vi "DOCK_AUDIT_MAIN.vi"() -> ()   [LabVIEW 2020]
uses:
  DOCK_AUDIT/MAIN/DOCK_header_data_display.ctl
  DOCK_AUDIT/FGV/error_buffer/FGV_DOCK_error_buffer.ctl
  DOCK_AUDIT/ini/typedef/DOCK_all_config_info.ctl
  DOCK_AUDIT/ini/typedef/DOCK_main_ini_file.ctl
  DOCK_AUDIT/queues/typedef/DOCK_queue_refnums.ctl
  DOCK_AUDIT/queues/typedef/DOCK_MAIN_queue_element.ctl
  DOCK_AUDIT/MAIN/DOCK_MAIN_sequence_state.ctl
  DOCK_AUDIT/queues/typedef/DOCK_SCANNER_queue_element.ctl
  DOCK_AUDIT/SCANNER/DOCK_SCANNER_sequence_state.ctl
  DOCK_AUDIT/queues/typedef/DOCK_PRINTER_queue_element.ctl
  DOCK_AUDIT/PRINTER/DOCK_PRINTER_sequence_state.ctl
  DOCK_AUDIT/FGV/SQL_connection/FGV_DOCK_SQL_connection.ctl
  DOCK_AUDIT/FGV/login/DOCK_login_refnums.ctl
  DOCK_AUDIT/FGV/login/FGV_DOCK_login.ctl
  DOCK_AUDIT/FGV/DOCK_status_display/FGV_DOCK_status_display.ctl
  DOCK_AUDIT/FGV/DOCK_records_display/FGV_DOCK_records_display.ctl
  DOCK_AUDIT/FGV/DOCK_records_display/DOCK_references.ctl
  DOCK_AUDIT/FGV/controls_state/FGV_DOCK_controls_state.ctl
  DOCK_AUDIT/FGV/controls_state/FGV_DOCK_controls_state_refnums.ctl
  DOCK_AUDIT/FGV/DOCK_batch_ID_buffer/FGV_DOCK_batch_ID_buffer.ctl
  DOCK_AUDIT/FGV/DOCK_multistate_indicator/FGV_DOCK_multistate_indicator.ctl
  DOCK_AUDIT/FGV/DOCK_REPORT_records_display/FGV_DOCK_REPORT_records_display.ctl
  DOCK_AUDIT/FGV/DOCK_REPORT_records_display/DOCK_REPORT_references.ctl
  DOCK_AUDIT/FGV/DOCK_REPORT_status_display/FGV_DOCK_REPORT_status_display.ctl
  DOCK_AUDIT/MAIN/DOCK_thread.ctl
  DOCK_AUDIT/ini/typedef/DOCK_reload_data.ctl
  DOCK_AUDIT/FGV/config_info/FGV_DOCK_config_info.ctl
  _misc/AULocalize/SubVIs/RegisterVI.vi
  <vilib>/Instr/_visa.llb/VISA Configure Serial Port (Instr).vi
  _misc/AULocalize/SubVIs/Get Localized Phrase Compact Interface 1D.vi
  _misc/AULocalize/SubVIs/Get Localized Phrase Compact Interface 0D.vi
panel:
  out "app_title":string caption="A603 - Dock Audit"
  in  "reload_reference_data":bool
  in  "print_label_test":bool
  out "reload_active?":bool
  out "reload_batch_size":u16 caption="Размер партии:"
  out "reload_part_number":string caption="Номер партии:"
  in  "printer_send_label":bool
  in  "printer_send_template":bool
  out "current_batch_count":u16 caption="В текущей партии:"
  out "batch_active?":bool
  out "PRINTER_connection_indicator_global":bool caption="Статус подключения принтера:"
  in  "DOCK_start_finish_batch":bool
  in  "BATCH_SIZE_selector":u16(ring)=30 caption="Размер партии:" items=["36"=36, "30"=30, "10"=10, "6"=6, "1"=1]
  in  "REFERENCE_selector":u16(ring) caption="Тип детали:" items=["CMFB", "VESTA"]
  in  "USER_login_logout":bool
  out "SQL_connection_indicator_global":bool caption="Статус подключения SQL:"
  out "ERROR_indicator_global":bool caption="Статус программы:"
  out "current_access_level":i32 caption="Уровень доступа:"
  out "current_username":string="-" caption="Вход под ID:"
  in  "main_tab":enum32{"Dock Audit", "Current Batch", "Errors"}(tab)=enum."Errors"
  out "gear_serial_display":string
  in  "gear_NOK":bool
  in  "gear_OK":bool
  in  "DOCK_clear_gear_data":bool
  out "DOCK_multistate_indicator":bool=TRUE
  in  "DOCK_read_gear_data":bool
  in  "DOCK_records":i32(listbox)=-1
  out "DOCK_SQL_status":string="READ BATCH SIZE LIST - OK\nExecuted SQL statement: SELECT DISTINCT BATCH_SIZE FROM DOCK_AUDIT_BATCH_SIZE ORDER BY BATCH_SIZE DESC"
  in  "DOCK_gear_serial":string caption="Номер детали:"
  out "batch_code_display":string
  out "DOCK_header_data_display":T1
  out "input_header":string caption="Вход"
  out "gear_info_summary_header":string caption="Информация о детали"
  in  "REPORT_clear":bool
  in  "REPORT_records":i32(listbox)=-1
  out "DOCK_REPORT_SQL_status":string="READ BATCH SIZE LIST - OK\nExecuted SQL statement: SELECT DISTINCT BATCH_SIZE FROM DOCK_AUDIT_BATCH_SIZE ORDER BY BATCH_SIZE DESC"
  in  "REPORT_reload":bool
  out "REPORT_current_batch":string
  in  "ERROR_records":i32(listbox)=-1
  in  "ERROR_clear":bool
  out "ERROR_indicator_tab":bool
  in  "STOP":bool=TRUE
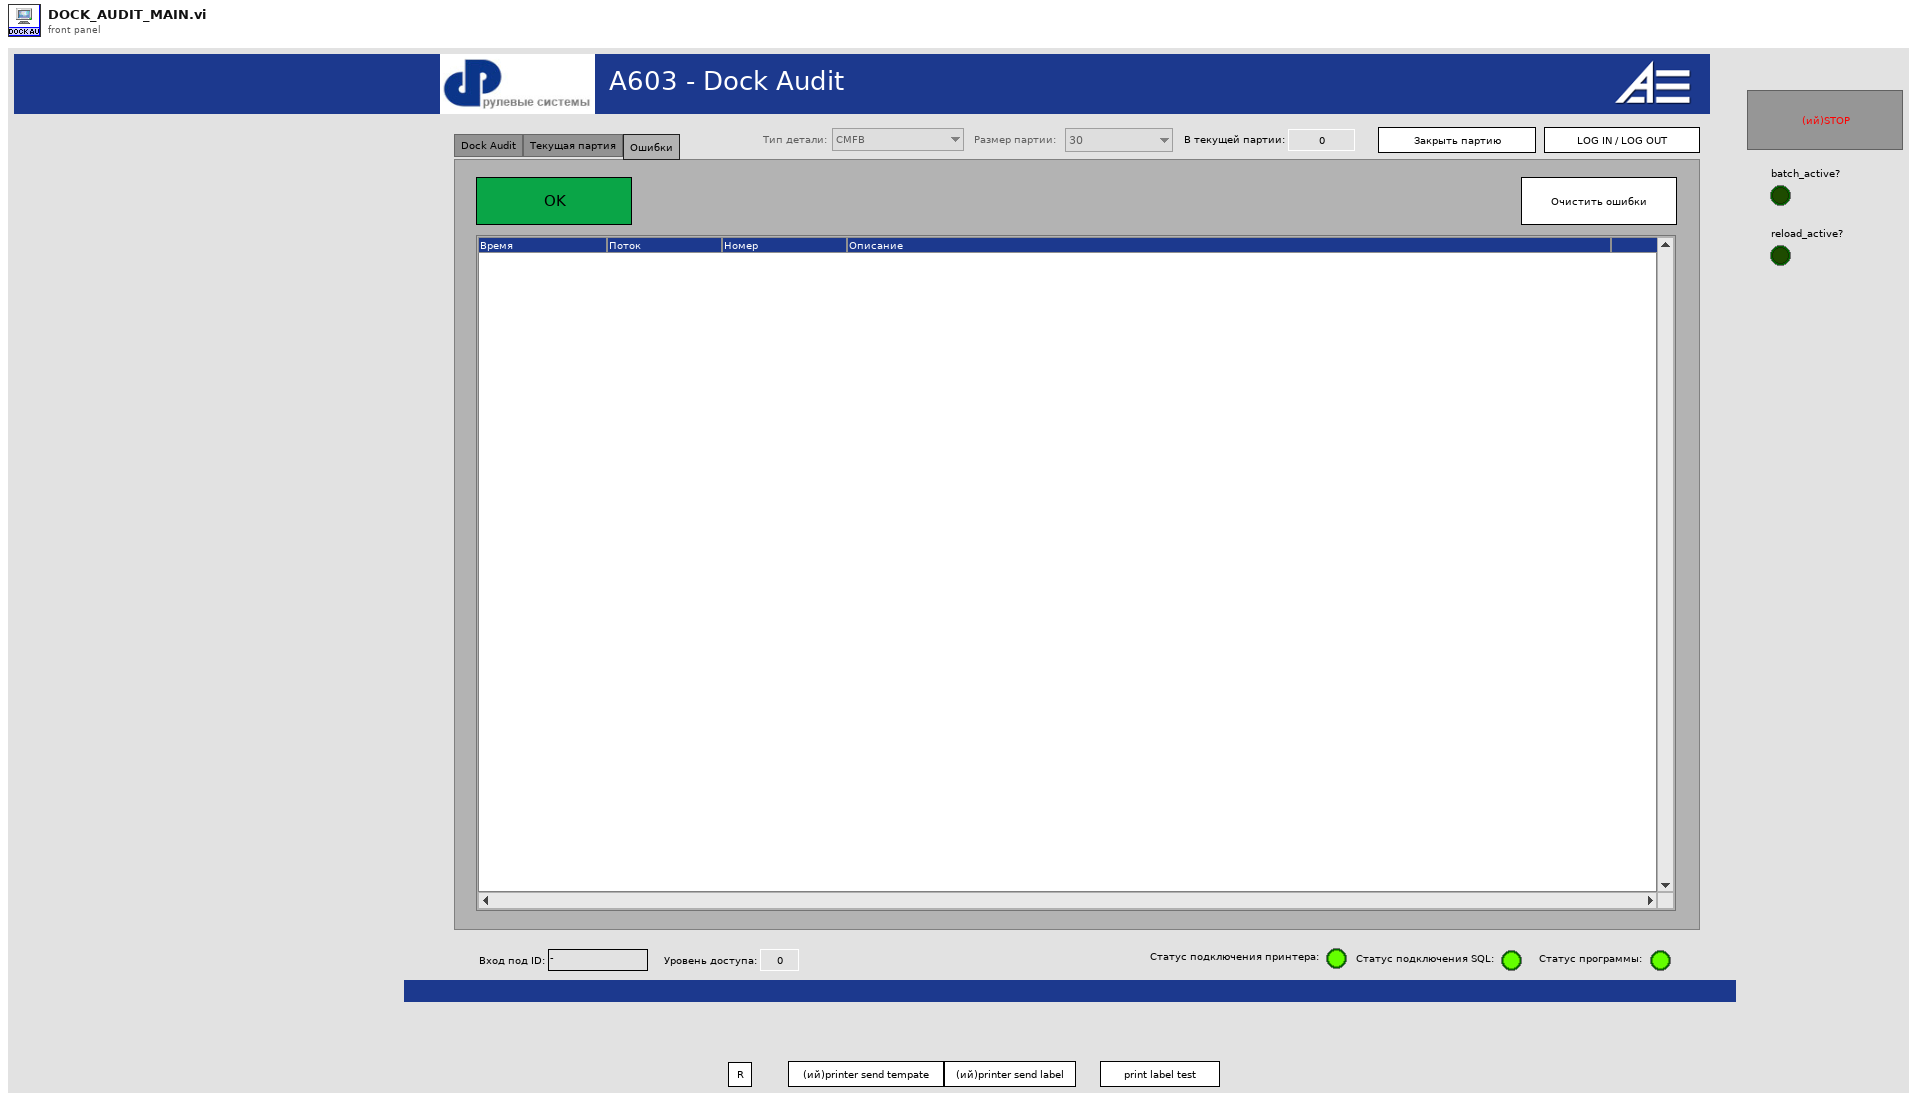
[diagram p1: front panel]
types:
  T1 = typedef "DOCK_header_data_display.ctl" = cluster{"ID":string, "creation_time":string, "last_station":string, "last_status":string, "pinion_serial":string, "batch_code":string}
  T2 = typedef "FGV_DOCK_REPORT_status_display.ctl" = enum16{"initialize", "display", "clear"}
  T3 = typedef "DOCK_REPORT_references.ctl" = cluster{"front_panel_reference":refnum<vi>, "SQL_listbox_reference":refnum<vi>}
  T4 = typedef "FGV_DOCK_REPORT_records_display.ctl" = enum16{"initialize", "set_cbatch_code", "set_records", "display", "clear", "get_all_info"}
  T5 = typedef "FGV_DOCK_multistate_indicator.ctl" = enum16{"initialize", "login", "logout", "start_batch", "finish_batch", "gear_OK", "gear_NOK", "gear_clear", "translate", "error", "error_clear"}
  T6 = typedef "DOCK_MAIN_queue_element.ctl" = cluster{"state":T7, "variable":variant}
  T7 = typedef "DOCK_MAIN_sequence_state.ctl" = enum16{"initialize", "get_next_state", "USER_login", "USER_logout", "read_reference_list", "read_batch_size_list", "change_reference", "start_batch", "reload_batch", "finish_batch?", "finish_batch", "preread_gear_data_check", "read_gear_data", "refresh_gear_data", "save_gear_to_batch", "clear_gear_data", "print_label", "report_get", "error", "stop"}
  T8 = typedef "FGV_DOCK_batch_ID_buffer.ctl" = enum16{"initialize", "buffer_batch_ID", "get_ID_for_batch"}
  T9 = typedef "FGV_DOCK_controls_state_refnums.ctl" = cluster{"REFERENCE_selector":refnum<vi>, "BATCH_SIZE_selector":refnum<vi>, "DOCK_start_finish_batch":refnum<vi>, "gear_OK":refnum<vi>, "gear_NOK":refnum<vi>, "reload_part_number":refnum<vi>, "reload_batch_size":refnum<vi>, "menu_bar":refnum<k9>}
  T10 = typedef "FGV_DOCK_controls_state.ctl" = enum16{"initialize", "login_event", "translation_event", "batch_event", "reload_event", "gear_event", "gear_saved_event", "gear_in_another_batch_event", "gear_in_current_batch_event", "NOK_ref_gear_event", "NOK_station_gear_event", "get_gear_loaded_status"}
  T11 = typedef "DOCK_references.ctl" = cluster{"front_panel_reference":refnum<vi>, "SQL_listbox_reference":refnum<vi>, "DOCK_header_data_display":refnum<vi>}
  T12 = typedef "FGV_DOCK_records_display.ctl" = enum16{"initialize", "set_reference_data", "set_serial", "set_header", "set_operations", "set_results", "set_batches", "get_reference_data", "get_part_number_ref", "get_serial", "get_batch_code", "get_gear_ID", "get_operation_IDs", "toggle_results", "show_all_results", "hide_all_results", "display", "clear"}
  T13 = typedef "FGV_DOCK_status_display.ctl" = enum16{"initialize", "display", "clear"}
  T14 = typedef "DOCK_PRINTER_sequence_state.ctl" = enum16{"initialize", "get_next_state", "send", "keep_alive", "error", "stop"}
  T15 = typedef "FGV_DOCK_login.ctl" = enum16{"initialize", "start_login_read", "end_login_read", "login", "logout", "get_login_info"}
  T16 = typedef "DOCK_login_refnums.ctl" = cluster{"current_username":refnum<vi>, "current_access_level":refnum<vi>}
  T17 = typedef "DOCK_SCANNER_sequence_state.ctl" = enum16{"initialize", "get_next_state", "read", "error", "stop"}
  T18 = typedef "FGV_DOCK_SQL_connection.ctl" = enum16{"initialize", "connect", "read_tables", "read_columns", "SELECT", "INSERT", "UPDATE", "DELETE", "EXEC + headers", "EXEC", "TRANSACTION", "connection_active?", "disconnect"}
  T19 = typedef "DOCK_all_config_info.ctl" = cluster{"main_ini_file":T20, "SQL Password":string, "PRINTER Label":string, "PRINTER Template":string, "Last Label":string, "queue_refnums":T21}
  T20 = typedef "DOCK_main_ini_file.ctl" = cluster{"SQL Driver":string, "SQL Server":string, "SQL Database":string, "SQL UID":string, "Reference table":string, "Reference history":string, "Archivisation CFG table":string, "Archivisation CFG history":string, "User table":string, "User history":string, "default language":string, "SCANNER COM port":u16, "SCANNER Baud rate":u32, "SCANNER Data bits":u16, "SCANNER Pairity":enum16{"None", "Odd", "Even", "Mark", "Space"}, "SCANNER Stop bits":u16, "SCANNER Flow control":u16, "SCANNER Termination char":u8, "PRINTER PC port":u16, "PRINTER IP":string, "PRINTER port":u16, "PRINTER Keep alive timer [ms]":i32, "logout timeout [ms]":i32}
  T21 = typedef "DOCK_queue_refnums.ctl" = cluster{"MAIN_queue":refnum<queue>, "SCANNER_queue":refnum<queue>, "SCANNER_login":refnum<queue>, "PRINTER_queue":refnum<queue>}
  T22 = typedef "FGV_DOCK_error_buffer.ctl" = enum16{"initialize", "clear", "display", "get_status"}
  T23 = typedef "DOCK_PRINTER_queue_element.ctl" = cluster{"state":T14, "variable":variant}
  T24 = typedef "DOCK_SCANNER_queue_element.ctl" = cluster{"state":T17, "variable":variant}
  T25 = typedef "DOCK_reload_data.ctl" = cluster{"batch_ID":string, "batch_code":string, "declared_size":u16, "current_size":u16, "part_number":string}
  T26 = typedef "DOCK_thread.ctl" = enum16{"MAIN", "SCANNER", "PRINTER"}
  T27 = typedef "FGV_DOCK_config_info.ctl" = enum16{"initialize", "set", "set_last_label", "get"}
  T28 = enum32{"Dock Audit", "Current Batch", "Errors"}[]
  T29 = typedef "DOCK_PRINTER_label_fields.ctl" = cluster{"packaging_date":string, "quantity":string, "part_number":string, "part_name":string, "PSW_number":string, "batch_number":string, "AUSS, TS":string, "packager":string, "barcode":string}
  T30 = enum8{"Enabled", "Disabled", "Disabled and Grayed Out"}
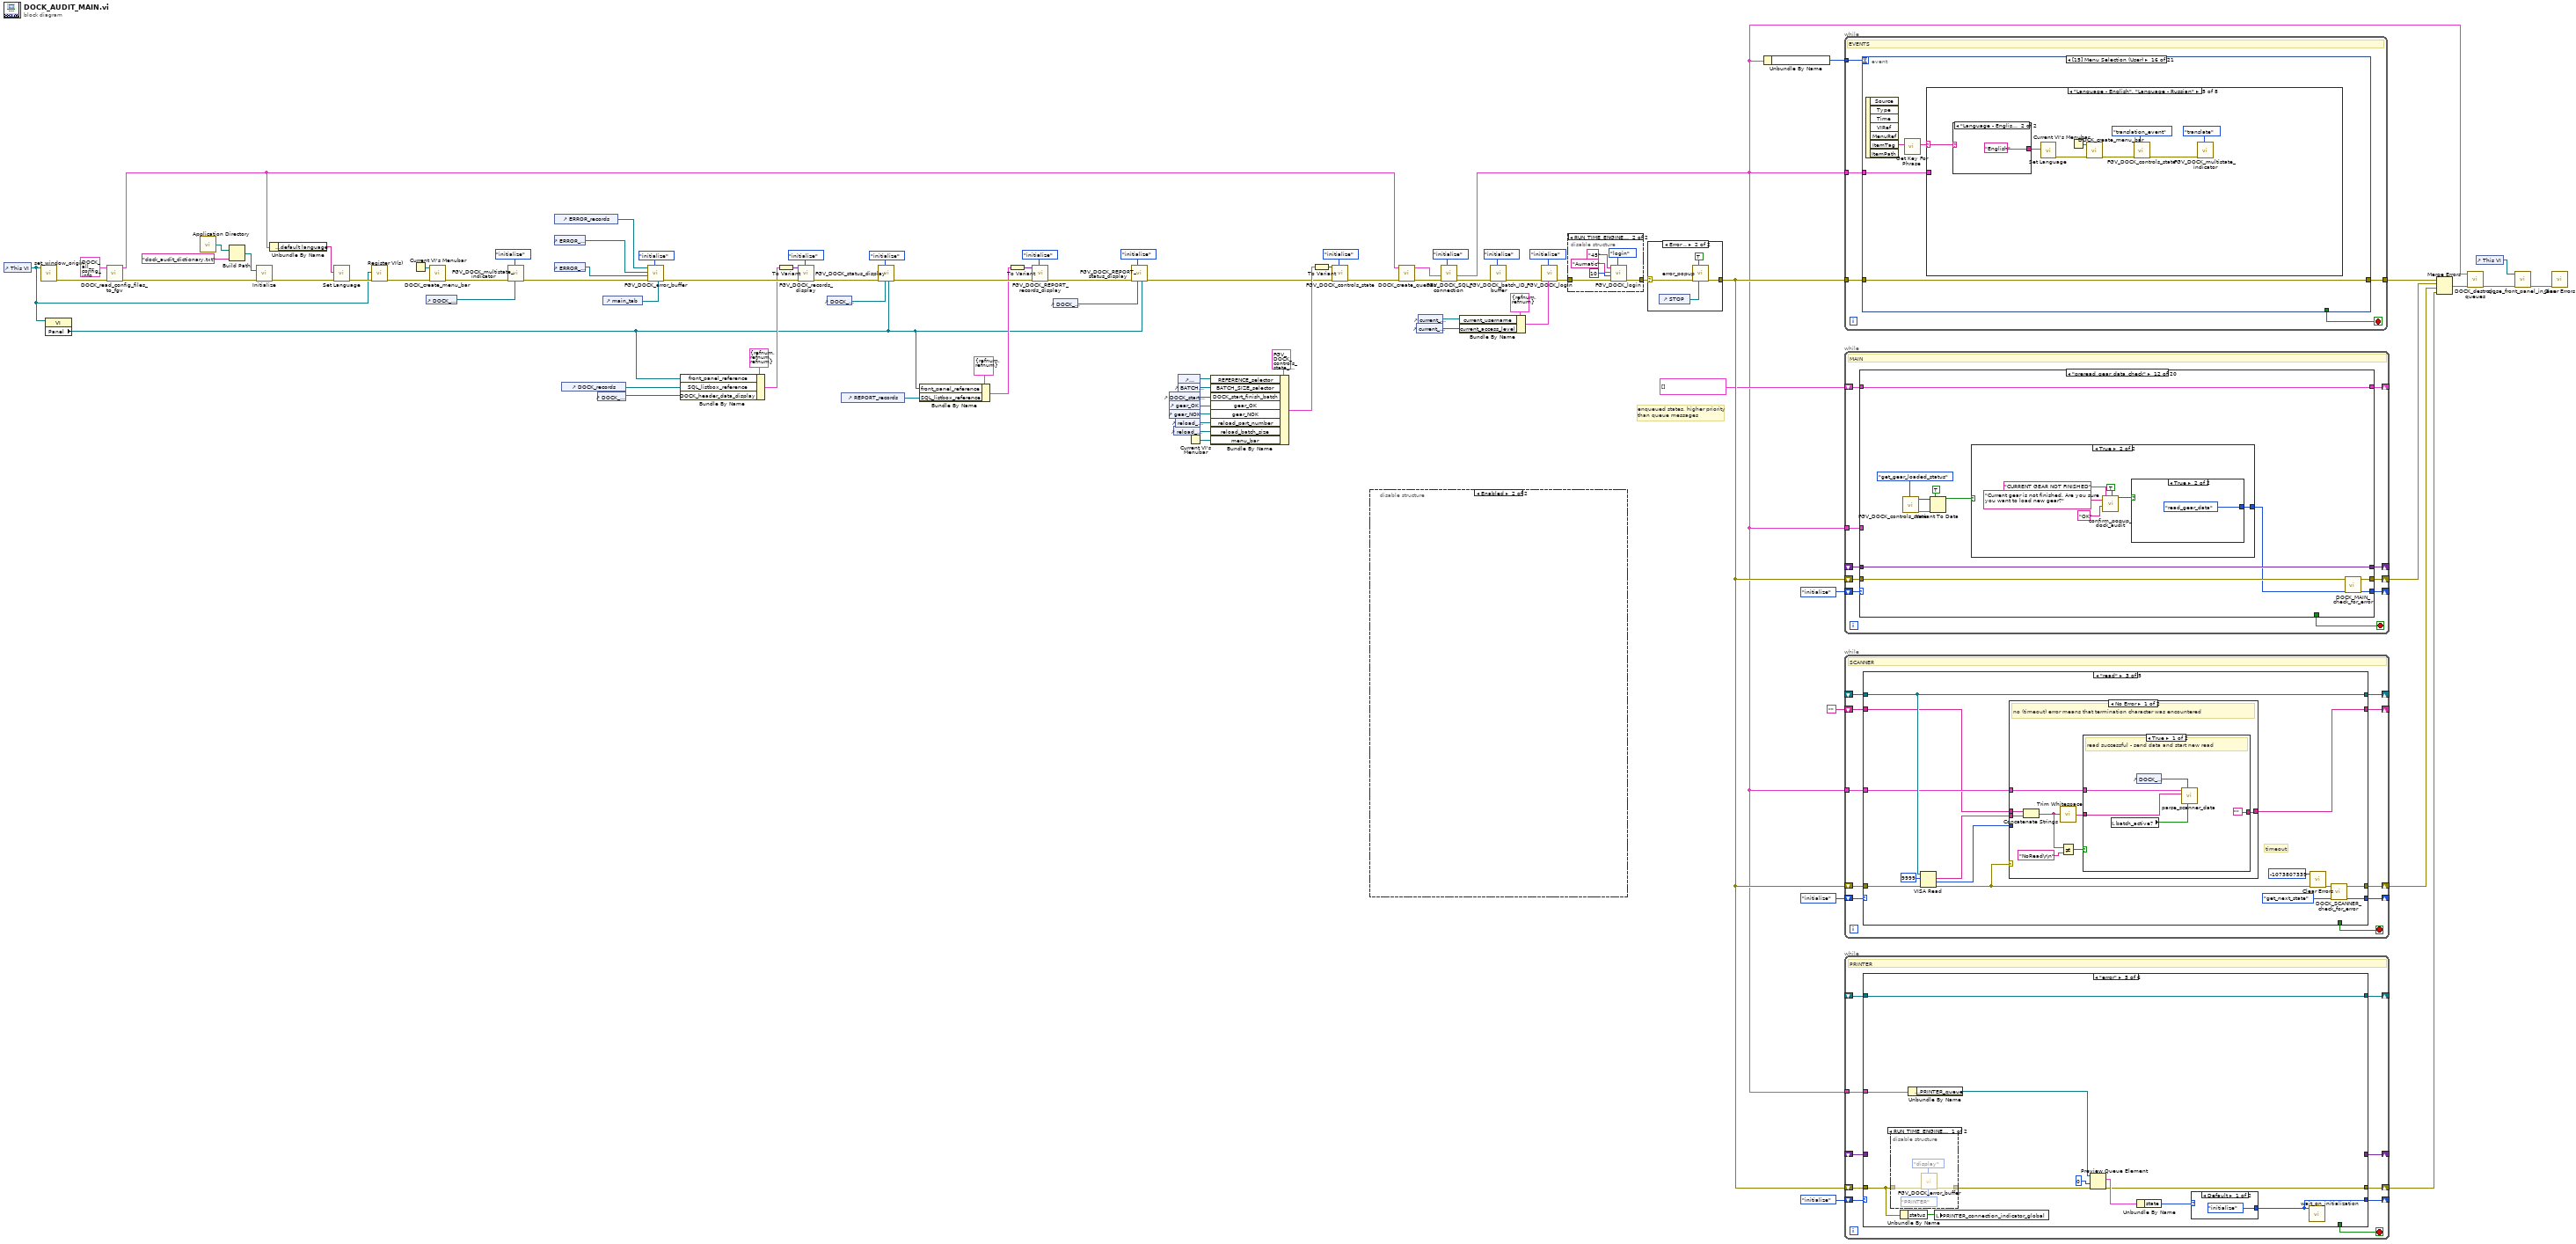
[diagram p0: block diagram]
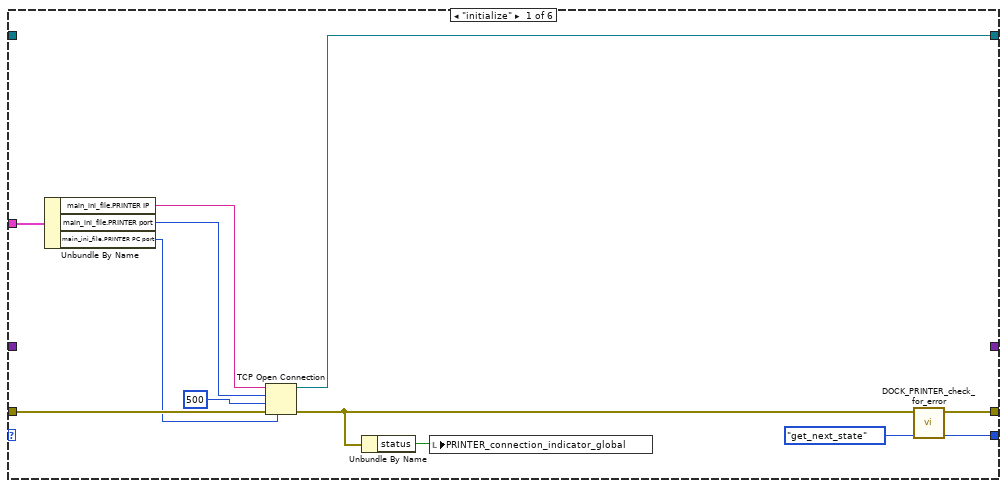
[diagram p3: hidden frame]
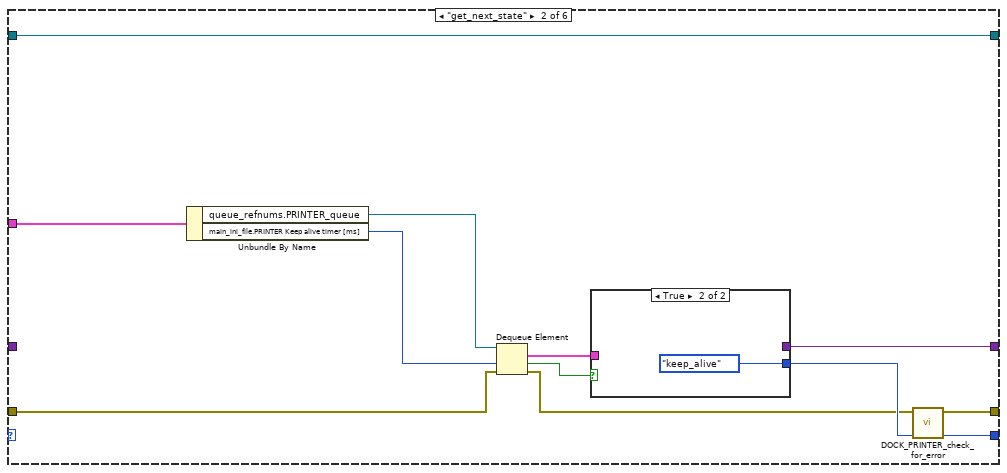
[diagram p4: hidden frame]
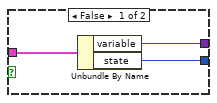
[diagram p5: hidden frame]
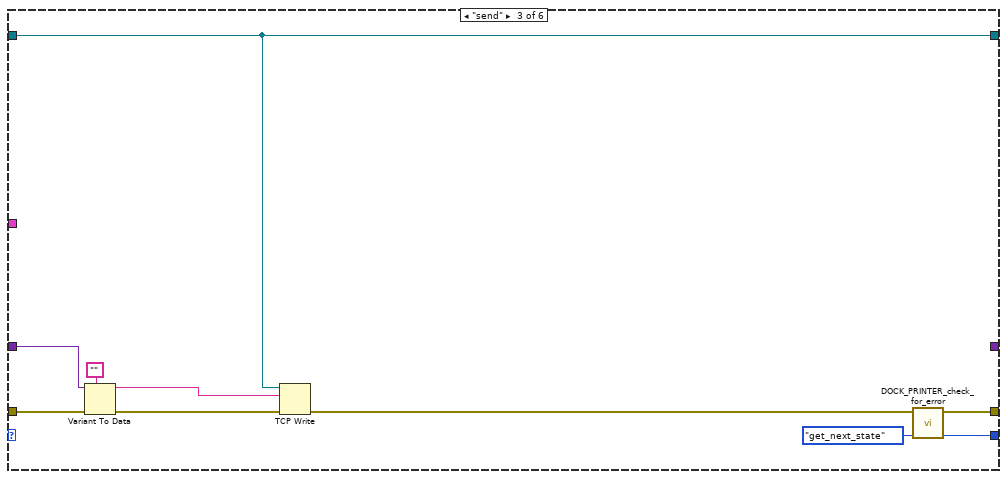
[diagram p6: hidden frame]
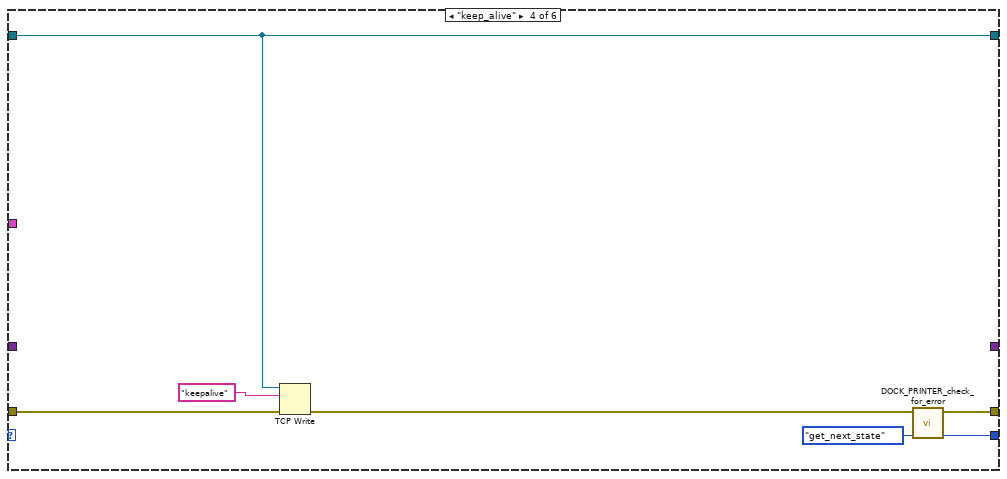
[diagram p7: hidden frame]
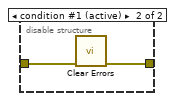
[diagram p8: hidden frame]
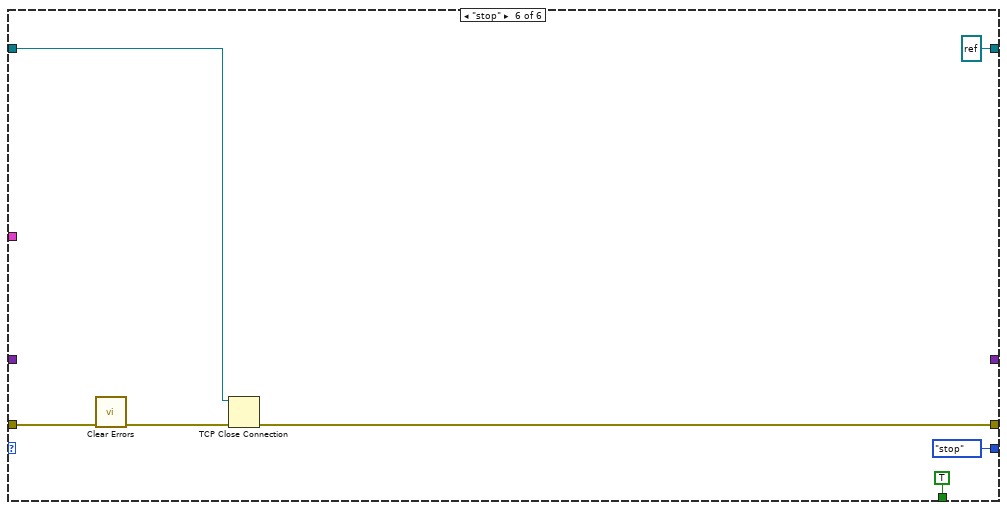
[diagram p10: hidden frame]
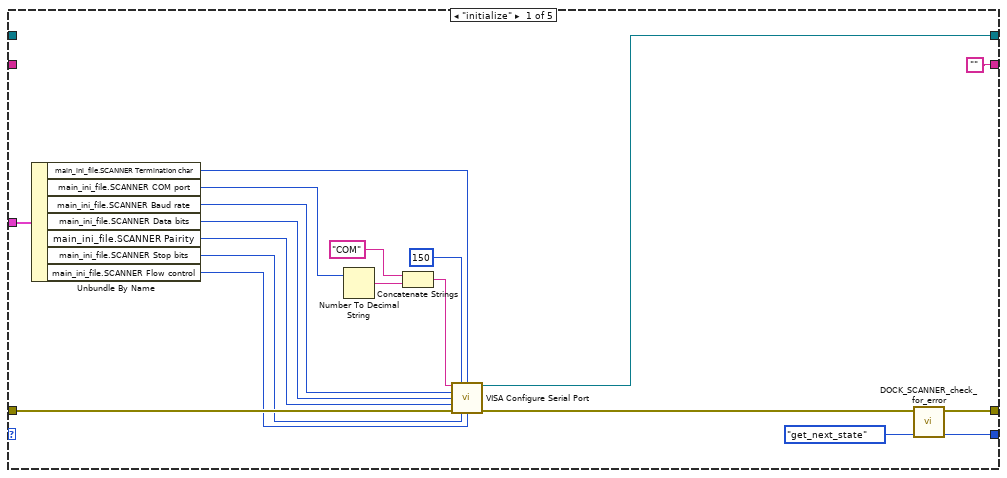
[diagram p11: hidden frame]
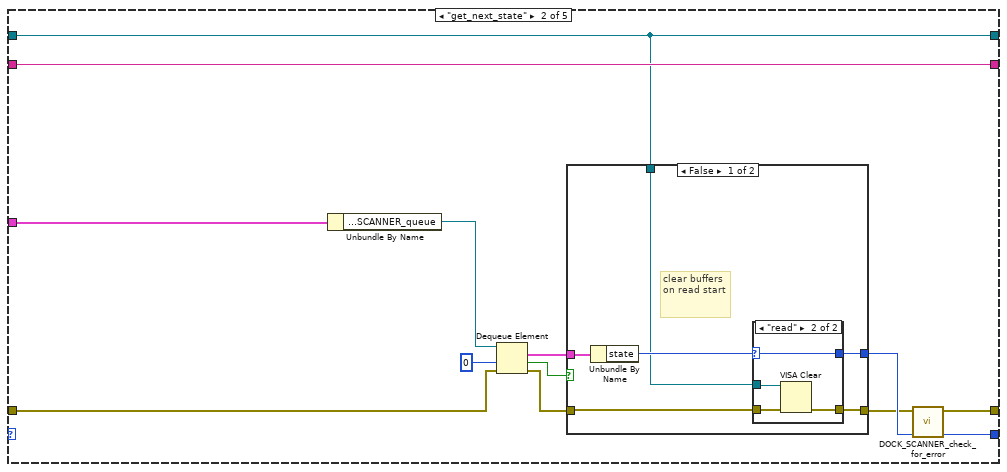
[diagram p12: hidden frame]
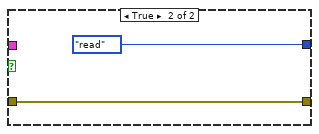
[diagram p14: hidden frame]
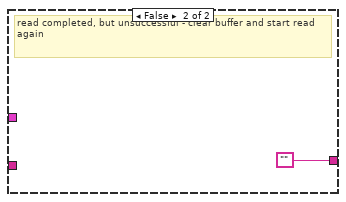
[diagram p15: hidden frame]
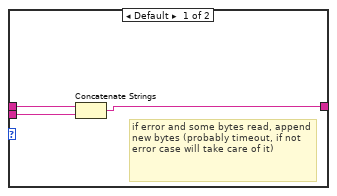
[diagram p17: hidden frame]
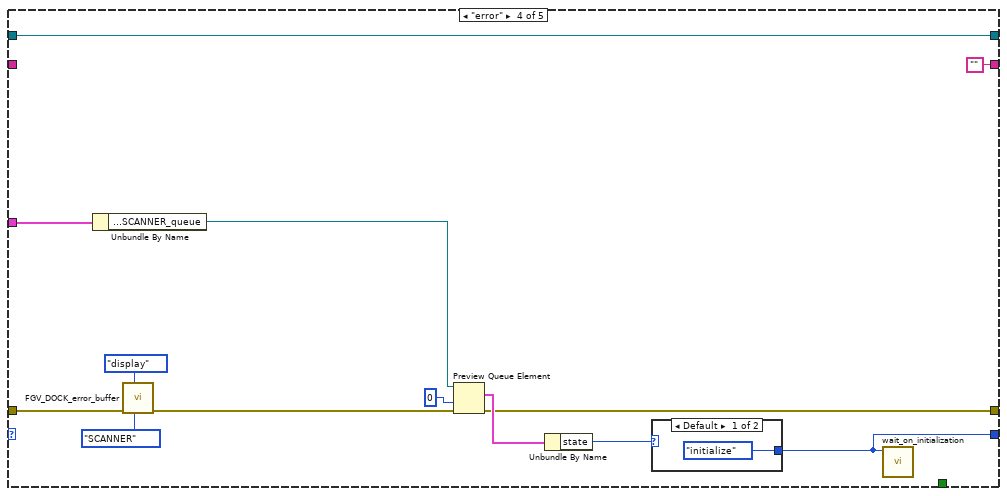
[diagram p18: hidden frame]
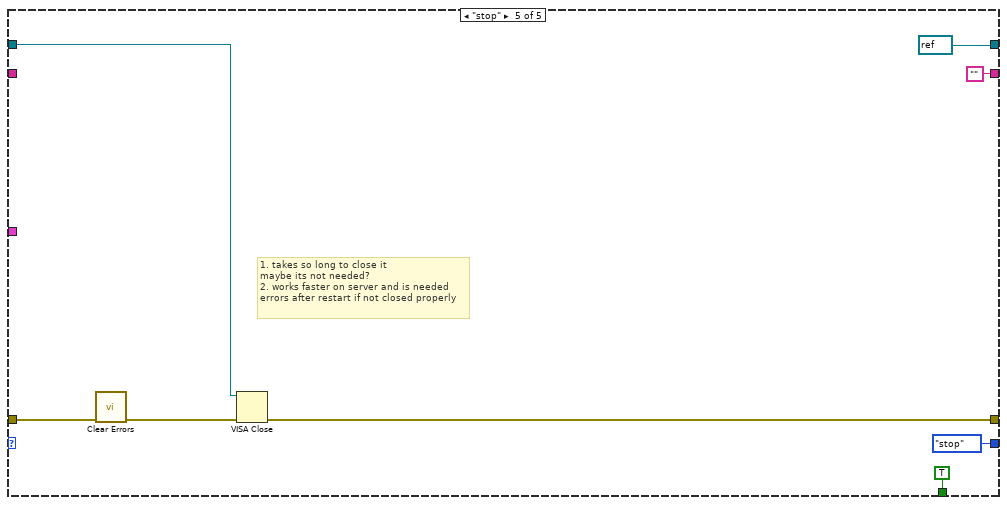
[diagram p20: hidden frame]
diagram:
  # "enqueued states, higher priority\nthan queue messages"
  n1 = control-ref of="This VI"() -> (w5:refnum<vi>)
  n2 = call "set_window_origin.vi"("this_vi_reference"=w5) -> ("error_out"=w11:errorcluster)  [unwired: 10 in]
  n3 = property class="VI"(reference=w5) -> ("Panel"=w15:refnum<vi>)  [unwired: 1 in, 2 out]
  n4 = call "DOCK_read_config_files_to_fgv.vi"("error_in"=w11, "all_config_info_in"=T19 {"main_ini_file"={"SQL Driver"="", "SQL Server"="", "SQL Database"="", "SQL UID"="", "Reference table"="", "Reference history"="", "Archivisation CFG table"="", "Archivisation CFG history"="", "User table"="", "User history"="", "default language"="", "SCANNER COM port"=0, "SCANNER Baud rate"=0, "SCANNER Data bits"=0, "SCANNER Pairity"=enum."None", "SCANNER Stop bits"=10, "SCANNER Flow control"=0, "SCANNER Termination char"=0, "PRINTER PC port"=0, "PRINTER IP"="", "PRINTER port"=0, "PRINTER Keep alive timer [ms]"=0, "logout timeout [ms]"=0}, "SQL Password"="", "PRINTER Label"="", "PRINTER Template"="", "Last Label"="", "queue_refnums"={"MAIN_queue"=refnum, "SCANNER_queue"=refnum, "SCANNER_login"=refnum, "PRINTER_queue"=refnum}}) -> ("error_out"=w4:errorcluster, "all_config_info_out"=w3:T19)  [unwired: 8 in]
  n5 = call <vilib>:"Application Directory.vi"() -> ("Application Directory"=w10:path)
  n6 = Build Path(base path=w10, name or relative path="dock_audit_dictionary.txt") -> (appended path=w2:path)
  n7 = call "Initialize.vi"("Dictionary File Path"=w2, "error in"=w4) -> ("error out"=w8:errorcluster)  [unwired: 8 in, 5 out]
  n8 = Unbundle By Name(w3) -> ("main_ini_file.default language"=w6:string)
  n9 = call "Set Language.vi"("error in"=w8, "Target Language (current lang)"=w6) -> ("error out"=w7:errorcluster)  [unwired: 8 in, 1 out]
  n10 = call-poly "Register VI(s).vi"("error in"=w7, "VI Ref"=w5) -> ("error out"=w1:errorcluster)  [unwired: 8 in, 1 out]
  n11 = Current VI's Menubar() -> (w13:refnum<k9>)
  n12 = control-ref of="DOCK_multistate_indicator"() -> (w34:refnum<vi>)
  n13 = call "DOCK_create_menu_bar.vi"("error_in"=w1, "menu_bar_refnum"=w13) -> ("error_out"=w12:errorcluster)  [unwired: 9 in]
  n14 = call "FGV_DOCK_multistate_indicator.vi"("boolean_indicator_refnum"=w34, "options"=FGV_DOCK_multistate_indicator."initialize", "error_in"=w12) -> ("error_out"=w32:errorcluster)  [unwired: 8 in]
  n15 = control-ref of="ERROR_records"() -> (w82:refnum<vi>)
  n16 = control-ref of="ERROR_indicator_tab"() -> (w81:refnum<vi>)
  n17 = control-ref of="ERROR_indicator_global"() -> (w80:refnum<vi>)
  n18 = control-ref of="DOCK_records"() -> (w50:refnum<vi>)
  n19 = control-ref of="DOCK_header_data_display"() -> (w49:refnum<vi>)
  n20 = control-ref of="main_tab"() -> (w79:refnum<vi>)
  n21 = call "FGV_DOCK_error_buffer.vi"("main_tab"=w79, "option"=FGV_DOCK_error_buffer."initialize", "error_in"=w32, "error_indicator_global"=w80, "error_indicator_tab"=w81, "error_display_ref"=w82) -> ("error_out"=w56:errorcluster)  [unwired: 4 in, 1 out]
  n22 = Bundle By Name(cluster=T11 {"front_panel_reference"=refnum, "SQL_listbox_reference"=refnum, "DOCK_header_data_display"=refnum} ("REWORK_references"), "front_panel_reference"=w15, "SQL_listbox_reference"=w50, "DOCK_header_data_display"=w49) -> (w51:T11)
  n23 = To Variant(anything=w51) -> (Variant=w53:variant)
  n24 = call "FGV_DOCK_records_display.vi"("options"=FGV_DOCK_records_display."initialize", "error_in"=w56, "input"=w53) -> ("error_out"=w55:errorcluster)  [unwired: 7 in, 1 out]
  n25 = control-ref of="DOCK_SQL_status"() -> (w57:refnum<vi>)
  n26 = control-ref of="REPORT_records"() -> (w19:refnum<vi>)
  n27 = call "FGV_DOCK_status_display.vi"("front_panel_reference"=w15, "status_display_reference"=w57, "options"=FGV_DOCK_status_display."initialize", "error_in"=w55) -> ("error_out"=w24:errorcluster)  [unwired: 7 in]
  n28 = Bundle By Name(cluster=T3 {"front_panel_reference"=refnum, "SQL_listbox_reference"=refnum} ("REWORK_references"), "front_panel_reference"=w15, "SQL_listbox_reference"=w19) -> (w20:T3)
  n29 = To Variant(anything=w20) -> (Variant=w21:variant)
  n30 = call "FGV_DOCK_REPORT_records_display.vi"("options"=FGV_DOCK_REPORT_records_display."initialize", "error_in"=w24, "input"=w21) -> ("error_out"=w18:errorcluster)  [unwired: 7 in, 1 out]
  n31 = control-ref of="DOCK_REPORT_SQL_status"() -> (w14:refnum<vi>)
  n32 = call "FGV_DOCK_REPORT_status_display.vi"("front_panel_reference"=w15, "status_display_reference"=w14, "options"=FGV_DOCK_REPORT_status_display."initialize", "error_in"=w18) -> ("error_out"=w17:errorcluster)  [unwired: 7 in]
  n33 = control-ref of="DOCK_start_finish_batch"() -> (w43:refnum<vi>)
  n34 = control-ref of="gear_OK"() -> (w42:refnum<vi>)
  n35 = control-ref of="gear_NOK"() -> (w41:refnum<vi>)
  n36 = control-ref of="reload_batch_size"() -> (w26:refnum<vi>)
  n37 = control-ref of="reload_part_number"() -> (w27:refnum<vi>)
  n38 = control-ref of="REFERENCE_selector"() -> (w45:refnum<vi>)
  n39 = control-ref of="BATCH_SIZE_selector"() -> (w44:refnum<vi>)
  n40 = Current VI's Menubar() -> (w25:refnum<k9>)
  n41 = Bundle By Name(cluster=T9 {"REFERENCE_selector"=refnum, "BATCH_SIZE_selector"=refnum, "DOCK_start_finish_batch"=refnum, "gear_OK"=refnum, "gear_NOK"=refnum, "reload_part_number"=refnum, "reload_batch_size"=refnum, "menu_bar"=refnum} ("control_refnums"), "REFERENCE_selector"=w45, "BATCH_SIZE_selector"=w44, "DOCK_start_finish_batch"=w43, "gear_OK"=w42, "gear_NOK"=w41, "reload_part_number"=w27, "reload_batch_size"=w26, "menu_bar"=w25) -> (w39:T9)
  n42 = To Variant(anything=w39) -> (Variant=w40:variant)
  n43 = call "FGV_DOCK_controls_state.vi"("options"=FGV_DOCK_controls_state."initialize", "error_in"=w17, "input"=w40) -> ("error_out"=w48:errorcluster)  [unwired: 7 in, 1 out]
  n44 = disable-structure shown="Enabled" {
    frame Disabled {
    }
    frame Enabled {
    }
  }
  n45 = call "DOCK_create_queues.vi"("error_in"=w48, "all_config_info_in"=w3) -> ("error_out"=w75:errorcluster, "all_config_info_out"=w76:T19)  [unwired: 8 in]
  n46 = control-ref of="current_access_level"() -> (w63:refnum<vi>)
  n47 = control-ref of="current_username"() -> (w64:refnum<vi>)
  n48 = call "FGV_DOCK_SQL_connection.vi"("options"=FGV_DOCK_SQL_connection."initialize", "error_in"=w75, "all_config_info_in"=w76) -> ("error_out"=w37:errorcluster, "all_config_info_out"=w29:T19)  [unwired: 4 in, 3 out]
  n49 = Bundle By Name(cluster=T16 {"current_username"=refnum, "current_access_level"=refnum} ("login_refnums"), "current_username"=w64, "current_access_level"=w63) -> (w65:T16)
  n50 = call "FGV_DOCK_batch_ID_buffer.vi"("options"=FGV_DOCK_batch_ID_buffer."initialize", "error_in"=w37) -> ("error_out"=w36:errorcluster)  [unwired: 7 in, 2 out]
  n51 = call "FGV_DOCK_login.vi"("login_refnums"=w65, "options"=FGV_DOCK_login."initialize", "error_in"=w36) -> ("error_out"=w31:errorcluster)  [unwired: 4 in, 4 out]
  n52 = disable-structure shown="RUN_TIME_ENGINE==False" {
    disable-tunnel: w31 -> [w86 w88]
    disable-tunnel: [w86 w87] -> w30
    frame condition #0 {
    }
    frame condition #1 (active) {
      n53 = call "FGV_DOCK_login.vi"("options"=FGV_DOCK_login."login", "error_in"=w88, "access_level_in"=10, "username_in"="Aumatic", "ID_in"="45") -> ("error_out"=w87:errorcluster)  [unwired: 2 in, 4 out]
    }
  }
  n54 = case shown="Error .." w30 {
    selector: w30 -> [w93 w96]
    tunnel: [w93 w97] -> w59
    frame No Error {
    }
    frame Error {
      n55 = control-ref of="STOP"() -> (w95:refnum<vi>)
      n56 = call "error_popup.vi"("STOP_button_reference"=w95, "EXIT App If Error? (F)"=TRUE, "error_in"=w96) -> ("error_out"=w97:errorcluster)  [unwired: 8 in]
    }
  }
  n57 = Unbundle By Name(w29) -> ("main_ini_file.logout timeout [ms]"=w28:i32)
  n58 = while {
    tunnel: w59 -> [w100]
    tunnel: [w102] -> w73
    tunnel: w29 -> [w99]
    tunnel: w28 -> [w98]
    stop <- w101 stop-if-true
    # "EVENTS"
    n59 = event shown="[15] Menu Selection (User)" {
      selector: _ -> [_ _ _ _ _ _ _ _ _ _ _ _ _ _ _ _ _ _ _ _ _]
      dyn-events: _ -> [_ _ _ _ _ _ _ _ _ _ _ _ _ _ _ _ _ _ _ _ _]
      timeout: w98 -> [_ _ _ _ _ _ _ _ _ _ _ _ _ _ _ _ _ _ _ _ _]
      tunnel: w100 -> [w103 w107 w141 w172 w177 w191 w209 w213 w220 w230 w233 w238 w247 w251 w256 w264 w344 w352 w358 w359 w366]
      tunnel: [w103 w110 w142 w172 w176 w190 w208 w212 w218 w229 w231 w236 w246 w250 w255 w264 w343 w351 w357 w359 w365] -> w102
      tunnel: [_ w109 _ _ _ _ _ _ _ _ _ _ _ _ _ _ _ _ _ _ _] -> w101
      tunnel: w99 -> [_ w105 w140 _ w175 w188 w207 w211 _ w228 w232 w237 w245 w249 _ w263 w345 w353 w356 _ w363]
      event "ERROR_clear": Value Change {
        n60 = event-data() -> ()  [unwired: 1 in, 6 out]
        n61 = call "FGV_DOCK_error_buffer.vi"("option"=FGV_DOCK_error_buffer."clear") -> ()  [unwired: 9 in, 2 out]
      }
      event "STOP": Value Change {
        n62 = event-data() -> ()  [unwired: 1 in, 6 out]
        n63 = disable-structure shown="RUN_TIME_ENGINE==True" {
          disable-tunnel: [w113 TRUE ("Result")] -> w108
          disable-tunnel: w107 -> [w112 w124]
          disable-tunnel: [w111 w124] -> w106
          frame condition #0 {
            n64 = case shown="No Error" w112 {
              selector: w112 -> [w118 w121]
              tunnel: [w119 TRUE ("Result")] -> w113
              tunnel: [w117 w121] -> w111
              frame No Error {
                n65 = call "confirm_popup.vi"("Warning(T)/Inf(F)"=TRUE, "error_in"=w118, "False Label"="No", "True Label"="Yes", "Message"="Are you sure you want to exit the application?") -> ("error_out"=w117:errorcluster, "Result"=w119:bool)  [unwired: 5 in]
              }
              frame Error {
              }
            }
          }
          frame condition #1 (active) {
          }
        }
        n66 = case shown="True" w108 {
          tunnel: w106 -> [w125 w131]
          tunnel: [w125 w127] -> w110
          tunnel: [FALSE TRUE] -> w109
          tunnel: w105 -> [_ w134]
          frame False {
          }
          frame True {
            n67 = Unbundle By Name(w134) -> ("queue_refnums.MAIN_queue"=w135:refnum<queue>, "queue_refnums.SCANNER_queue"=w137:refnum<queue>, "queue_refnums.PRINTER_queue"=w133:refnum<queue>)
            n68 = call <vilib>:"Clear Errors.vi"("error in (no error)"=w131) -> ("error out"=w132:errorcluster)  [unwired: 5 in, 1 out]
            n69 = Enqueue Element At Opposite End(queue=w133, element=T23 {"state"=enum."stop", "variable"=variant}, error in (no error)=w132) -> (error out=w138:errorcluster)  [unwired: 1 in, 2 out]
            n70 = Enqueue Element At Opposite End(queue=w137, element=T24 {"state"=enum."stop", "variable"=variant}, error in (no error)=w138) -> (error out=w136:errorcluster)  [unwired: 1 in, 2 out]
            n71 = Enqueue Element At Opposite End(queue=w135, element=T6 {"state"=enum."stop", "variable"=variant}, error in (no error)=w136) -> (error out=w127:errorcluster)  [unwired: 1 in, 2 out]
          }
        }
      }
      event "USER_login_logout": Value Change {
        n72 = event-data() -> ()  [unwired: 1 in, 6 out]
        n73 = call "FGV_DOCK_login.vi"("options"=FGV_DOCK_login."start_login_read", "error_in"=w141) -> ("error_out"=w146:errorcluster)  [unwired: 5 in, 4 out]
        n74 = local read "current_access_level"() -> (w145:i32)
        n75 = case shown="0" w145 {
          tunnel: [w153 w167] -> w147
          tunnel: w146 -> [w152 w165]
          tunnel: w140 -> [w151 w164]
          frame 0 {
            n76 = call "DOCK_LOGIN_scan_barcode.vi"("error_in"=w152, "all_config_info"=w151) -> ("error_out"=w150:errorcluster, "Canceled?"=w148:bool, "barcode"=w149:string)  [unwired: 7 in]
            n77 = case shown="True" w148 {
              tunnel: [w161 w162] -> w153
              tunnel: w150 -> [w158 w162]
              tunnel: w151 -> [w157 _]
              tunnel: w149 -> [w156 _]
              frame False {
                n78 = Unbundle By Name(w157) -> ("queue_refnums.MAIN_queue"=w160:refnum<queue>)
                n79 = To Variant(anything=w156) -> (Variant=w159:variant)
                n80 = Bundle By Name(cluster=T6 {"state"=enum."USER_login", "variable"=variant} ("element"), "variable"=w159) -> (w154:T6)
                n81 = Enqueue Element(queue=w160, element=w154, error in (no error)=w158) -> (error out=w161:errorcluster)  [unwired: 1 in, 2 out]
              }
              frame True {
              }
            }
          }
          frame Default {
            n82 = Unbundle By Name(w164) -> ("queue_refnums.MAIN_queue"=w166:refnum<queue>)
            n83 = Enqueue Element(queue=w166, element=T6 {"state"=enum."USER_logout", "variable"=variant}, error in (no error)=w165) -> (error out=w167:errorcluster)  [unwired: 1 in, 2 out]
          }
        }
        n84 = call "FGV_DOCK_login.vi"("options"=FGV_DOCK_login."end_login_read", "error_in"=w147) -> ("error_out"=w142:errorcluster)  [unwired: 5 in, 4 out]
      }
      event "current_access_level": Value Change {
        n85 = event-data() -> ("NewVal"=w170:i32)  [unwired: 1 in]
        n86 = case shown="Default" w170 {
          tunnel: [w173 w174] -> w171
          frame Default {
            w173 = T28 [enum."Errors"] items=["Dock Audit", "Current Batch", "Errors"]
          }
          frame 1..10 {
            w174 = T28 [enum."Dock Audit", enum."Current Batch", enum."Errors"] items=["Dock Audit", "Current Batch", "Errors"]
          }
        }
        n87 = control-ref of="main_tab"() -> (w168:refnum<vi>)
        n88 = control-ref of="This VI"() -> (w169:refnum<vi>)
        n89 = call "DOCK_show_hide_pages.vi"("This VI"=w169, "visible_pages"=w171, "main_tab_ref"=w168) -> ()  [unwired: 9 in]
      }
      event "main_tab": Value Change {
        n90 = event-data() -> ("NewVal"=w178:enum32{"Dock Audit", "Current Batch", "Errors"})  [unwired: 1 in]
        n91 = case shown="\"Current Batch\"" w178 {
          tunnel: w177 -> [w179 w183]
          tunnel: [w179 w182] -> w176
          tunnel: w175 -> [_ w181]
          frame Default {
          }
          frame "Current Batch" {
            n92 = local read "batch_code_display"() -> (w180:string)
            n93 = local write "REPORT_current_batch"(w180) -> ()
            n94 = Unbundle By Name(w181) -> ("queue_refnums.MAIN_queue"=w187:refnum<queue>)
            n95 = To Variant(anything=w180) -> (Variant=w185:variant)
            n96 = Bundle By Name(cluster=T6 {"state"=enum."report_get", "variable"=variant} ("element"), "variable"=w185) -> (w186:T6)
            n97 = Enqueue Element(queue=w187, element=w186, error in (no error)=w183) -> (error out=w182:errorcluster)  [unwired: 1 in, 2 out]
          }
        }
      }
      event "DOCK_start_finish_batch": Value Change {
        n98 = event-data() -> ()  [unwired: 1 in, 6 out]
        n99 = local read "batch_active?"() -> (w189:bool)
        n100 = case shown="False" w189 {
          tunnel: w191 -> [w195 w200]
          tunnel: [w192 w199] -> w190
          tunnel: w188 -> [w196 w201]
          frame False {
            n101 = Unbundle By Name(w196) -> ("queue_refnums.MAIN_queue"=w194:refnum<queue>)
            n102 = Enqueue Element(queue=w194, element=T6 {"state"=enum."start_batch", "variable"=variant}, error in (no error)=w195) -> (error out=w192:errorcluster)  [unwired: 1 in, 2 out]
          }
          frame True {
            n103 = Unbundle By Name(w201) -> ("queue_refnums.MAIN_queue"=w198:refnum<queue>)
            n104 = Enqueue Element(queue=w198, element=T6 {"state"=enum."finish_batch", "variable"=variant}, error in (no error)=w200) -> (error out=w199:errorcluster)  [unwired: 1 in, 2 out]
          }
        }
      }
      event "gear_OK": Value Change {
        n105 = event-data() -> ()  [unwired: 1 in, 6 out]
        n106 = Unbundle By Name(w207) -> ("queue_refnums.MAIN_queue"=w206:refnum<queue>)
        n107 = To Variant(anything=1) -> (Variant=w203:variant)
        n108 = Bundle By Name(cluster=T6 {"state"=enum."save_gear_to_batch", "variable"=variant} ("element"), "variable"=w203) -> (w204:T6)
        n109 = Enqueue Element(queue=w206, element=w204, error in (no error)=w209) -> (error out=w208:errorcluster)  [unwired: 1 in, 2 out]
      }
      event "REPORT_reload": Value Change {
        n110 = event-data() -> ()  [unwired: 1 in, 1 out]
        n111 = local read "REPORT_current_batch"() -> (w210:string)
        n112 = Unbundle By Name(w211) -> ("queue_refnums.MAIN_queue"=w217:refnum<queue>)
        n113 = To Variant(anything=w210) -> (Variant=w214:variant)
        n114 = Bundle By Name(cluster=T6 {"state"=enum."report_get", "variable"=variant} ("element"), "variable"=w214) -> (w215:T6)
        n115 = Enqueue Element(queue=w217, element=w215, error in (no error)=w213) -> (error out=w212:errorcluster)  [unwired: 1 in, 2 out]
      }
      event "REPORT_clear": Value Change {
        n116 = event-data() -> ()  [unwired: 1 in, 6 out]
        n117 = call "FGV_DOCK_REPORT_records_display.vi"("options"=FGV_DOCK_REPORT_records_display."clear", "error_in"=w220) -> ("error_out"=w219:errorcluster)  [unwired: 8 in, 1 out]
        n118 = call "FGV_DOCK_REPORT_status_display.vi"("options"=FGV_DOCK_REPORT_status_display."clear", "error_in"=w219) -> ("error_out"=w218:errorcluster)  [unwired: 9 in]
      }
      event "gear_NOK": Value Change {
        n119 = event-data() -> ()  [unwired: 1 in, 6 out]
        n120 = Unbundle By Name(w228) -> ("queue_refnums.MAIN_queue"=w227:refnum<queue>)
        n121 = To Variant(anything=2) -> (Variant=w224:variant)
        n122 = Bundle By Name(cluster=T6 {"state"=enum."save_gear_to_batch", "variable"=variant} ("element"), "variable"=w224) -> (w225:T6)
        n123 = Enqueue Element(queue=w227, element=w225, error in (no error)=w230) -> (error out=w229:errorcluster)  [unwired: 1 in, 2 out]
      }
      event "REFERENCE_selector": Value Change {
        n124 = event-data() -> ()  [unwired: 1 in, 6 out]
        n125 = Unbundle By Name(w232) -> ("queue_refnums.MAIN_queue"=w235:refnum<queue>)
        n126 = Enqueue Element(queue=w235, element=T6 {"state"=enum."change_reference", "variable"=variant}, error in (no error)=w233) -> (error out=w231:errorcluster)  [unwired: 1 in, 2 out]
      }
      event "reload_reference_data": Value Change {
        n127 = event-data() -> ()  [unwired: 1 in, 6 out]
        n128 = Unbundle By Name(w237) -> ("queue_refnums.MAIN_queue"=w240:refnum<queue>)
        n129 = Enqueue Element(queue=w240, element=T6 {"state"=enum."change_reference", "variable"=variant}, error in (no error)=w238) -> (error out=w236:errorcluster)  [unwired: 1 in, 2 out]
      }
      event "DOCK_read_gear_data": Value Change {
        n130 = event-data() -> ()  [unwired: 1 in, 6 out]
        n131 = local read "DOCK_gear_serial"() -> (w241:string)
        n132 = Unbundle By Name(w245) -> ("queue_refnums.MAIN_queue"=w248:refnum<queue>)
        n133 = To Variant(anything=w241) -> (Variant=w242:variant)
        n134 = Bundle By Name(cluster=T6 {"state"=enum."preread_gear_data_check", "variable"=variant} ("element"), "variable"=w242) -> (w243:T6)
        n135 = Enqueue Element(queue=w248, element=w243, error in (no error)=w247) -> (error out=w246:errorcluster)  [unwired: 1 in, 2 out]
      }
      event "DOCK_clear_gear_data": Value Change {
        n136 = event-data() -> ()  [unwired: 1 in, 6 out]
        n137 = Unbundle By Name(w249) -> ("queue_refnums.MAIN_queue"=w253:refnum<queue>)
        n138 = Enqueue Element(queue=w253, element=T6 {"state"=enum."clear_gear_data", "variable"=variant}, error in (no error)=w251) -> (error out=w250:errorcluster)  [unwired: 1 in, 2 out]
      }
      event "DOCK_records": Double Click {
        n139 = event-data() -> ("Row"=w254:i32)  [unwired: 1 in]
        n140 = To Variant(anything=w254) -> (Variant=w259:variant)
        n141 = call "FGV_DOCK_records_display.vi"("options"=FGV_DOCK_records_display."toggle_results", "error_in"=w256, "input"=w259) -> ("error_out"=w260:errorcluster)  [unwired: 7 in, 1 out]
        n142 = call "FGV_DOCK_records_display.vi"("options"=FGV_DOCK_records_display."display", "error_in"=w260) -> ("error_out"=w255:errorcluster)  [unwired: 8 in, 1 out]
      }
      event Menu Selection (User) {
        n143 = event-data() -> ("ItemTag"=w262:string)  [unwired: 1 in, 6 out]
        n144 = call "Get Key For Phrase.vi"("Phrase"=w262) -> ("Key"=w261:string)  [unwired: 9 in, 1 out]
        n145 = case shown="\"Language - English\", \"Language - Russian\"" w261 {
          selector: w261 -> [_ _ _ _ w322 _ _ _]
          tunnel: w263 -> [w269 w272 w298 w306 _ _ _ _]
          frame "Print Custom Label" {
            n146 = call "DOCK_PRINTER_print_label_manually.vi"() -> ("error_out"=w271:errorcluster, "do_printing?"=w268:bool, "label_fields_out"=w270:T29)  [unwired: 9 in]
            n147 = call "print_label.vi"("all_config_info"=w269, "error_in"=w271, "do_printing? (T)"=w268, "label_fields"=w270) -> ("error_out"=w265:errorcluster)  [unwired: 7 in]
            n148 = call "error_popup.vi"("EXIT App If Error? (F)"=FALSE, "error_in"=w265) -> ("error_out"=w266:errorcluster)  [unwired: 9 in]
            n149 = call <vilib>:"Clear Errors.vi"("error in (no error)"=w266) -> ()  [unwired: 5 in, 2 out]
          }
          frame "Reload Unfinished Batch" {
            n150 = call "DOCK_MAIN_choose_batch_to_reload.vi"() -> ("error_out"=w277:errorcluster, "declared_size"=w273:u16, "batch_code"=w274:string, "batch_ID"=w275:string, "Canceled?"=w276:bool)  [unwired: 7 in]
            n151 = case shown="False" w276 {
              tunnel: w277 -> [w293 _]
              tunnel: w275 -> [w287 _]
              tunnel: w274 -> [w286 _]
              tunnel: w273 -> [w279 _]
              tunnel: w272 -> [w285 _]
              frame False {
                n152 = Unbundle By Name(w285) -> ("queue_refnums.MAIN_queue"=w284:refnum<queue>)
                n153 = call "DOCK_MAIN_get_current_size_and_part_number.vi"("error_in"=w293, "batch_ID"=w287) -> ("error_out"=w290:errorcluster, "part_number"=w288:string, "current_size"=w278:u16)  [unwired: 7 in]
                n154 = Bundle By Name(cluster=T25 {"batch_ID"="", "batch_code"="", "declared_size"=0, "current_size"=0, "part_number"=""} ("main_ini_file"), "batch_ID"=w287, "batch_code"=w286, "declared_size"=w279, "current_size"=w278, "part_number"=w288) -> (w280:T25)
                n155 = To Variant(anything=w280) -> (Variant=w281:variant)
                n156 = call "FGV_DOCK_error_buffer.vi"("thread"=DOCK_thread."MAIN", "option"=FGV_DOCK_error_buffer."display", "error_in"=w290) -> ()  [unwired: 7 in, 2 out]
                n157 = Bundle By Name(cluster=T6 {"state"=enum."reload_batch", "variable"=variant} ("element"), "variable"=w281) -> (w282:T6)
                n158 = Enqueue Element(queue=w284, element=w282) -> ()  [unwired: 2 in, 3 out]
              }
              frame True {
              }
            }
          }
          frame "Send Template To Printer" {
            n159 = Unbundle By Name(w298) -> ("queue_refnums.PRINTER_queue"=w302:refnum<queue>, "PRINTER Template"=w297:string)
            n160 = To Variant(anything=w297) -> (Variant=w299:variant)
            n161 = Bundle By Name(cluster=T23 {"state"=enum."send", "variable"=variant} ("element"), "variable"=w299) -> (w300:T23)
            n162 = Enqueue Element(queue=w302, element=w300) -> ()  [unwired: 2 in, 3 out]
            n163 = call "message_popup.vi"("Message"="Template sent", "Title"="TEMPLATE SENT", "Button Label"="OK") -> ()  [unwired: 8 in, 1 out]
          }
          frame "Reprint Last Label" {
            n164 = Unbundle By Name(w306) -> ("queue_refnums.PRINTER_queue"=w307:refnum<queue>)
            n165 = call "FGV_DOCK_config_info.vi"("options"=FGV_DOCK_config_info."get") -> ("all_config_info_out"=w304:T19)  [unwired: 9 in, 1 out]
            n166 = Unbundle By Name(w304) -> ("Last Label"=w303:string)
            n167 = case shown="\"\"" w303 {
              selector: w303 -> [_ w311]
              tunnel: w307 -> [_ w315]
              frame "" {
                n168 = call "message_popup.vi"("Message"="Last Label is empty, label will not be printed.", "Title"="LABEL EMPTY", "Button Label"="OK") -> ()  [unwired: 8 in, 1 out]
              }
              frame Default {
                n169 = To Variant(anything=w311) -> (Variant=w312:variant)
                n170 = Bundle By Name(cluster=T23 {"state"=enum."send", "variable"=variant} ("element"), "variable"=w312) -> (w313:T23)
                n171 = Enqueue Element(queue=w315, element=w313) -> ()  [unwired: 2 in, 3 out]
              }
            }
          }
          frame "Language - English", "Language - Russian" {
            n172 = case shown="\"Language - English\", Default" w322 {
              tunnel: ["Russian" ("Target Language (current lang)") "English" ("Target Language (current lang)")] -> w323
              frame "Language - Russian" {
              }
              frame "Language - English", Default {
              }
            }
            n173 = call "Set Language.vi"("Target Language (current lang)"=w323) -> ("error out"=w320:errorcluster)  [unwired: 9 in, 1 out]
            n174 = Current VI's Menubar() -> (w321:refnum<k9>)
            n175 = call "DOCK_create_menu_bar.vi"("error_in"=w320, "menu_bar_refnum"=w321) -> ("error_out"=w317:errorcluster)  [unwired: 9 in]
            n176 = call "FGV_DOCK_controls_state.vi"("options"=FGV_DOCK_controls_state."translation_event", "error_in"=w317) -> ("error_out"=w316:errorcluster)  [unwired: 8 in, 1 out]
            n177 = call "FGV_DOCK_multistate_indicator.vi"("options"=FGV_DOCK_multistate_indicator."translate", "error_in"=w316) -> ()  [unwired: 9 in, 1 out]
          }
          frame "About" {
            n178 = disable-structure shown="Default" {
              disable-tunnel: [w332 w335] -> w328
              disable-tunnel: [w333 w335] -> w327
              frame condition #0 {
                n179 = vi-ref "get_exe_compilation_date.vi"() -> (w334:refnum<vi>)
                n180 = call-by-ref "?"(reference=w334) -> ("compilation_time"=w332:string, "compilation_date"=w333:string)  [unwired: 10 in, 3 out]
              }
              frame condition #1 (active) {
                n181 = call-poly "Get Localized Phrase Compact Interface.vi"("Key"="NOT COMPILED!" ("compilation_date")) -> ("Translated Phrase"=w335:string)
              }
            }
            n182 = call-poly "Get Localized Phrase Compact Interface.vi"("Key"="SQL Proxy Application\nMSG Assembly Line\nA603A00\n\nAumatic sp. z o.o.\nPilsudskiego 22\n32-050 Skawina\nPOLAND\n\nCOMPILATION DATE: %s\nCOMPILATION TIME: %s\nJakub Longa, 2020\n\n+48 (12) 256-77-90\naumatic.com" ("about_string")) -> ("Translated Phrase"=w326:string)
            n183 = Format Into String(format string=w326, w327, w328) -> (resulting string=w331:string)  [unwired: 2 in, 1 out]
            n184 = call "about_window.vi"("lines_to_bold"=i32[] [0, 1, 4, 9], "about_string"=w331) -> ()  [unwired: 9 in, 1 out]
          }
          frame "Exit" {
            n185 = property on="STOP" class="Bool (strict)"("Val(Sgnl)"=TRUE ("Value (Signaling)")) -> ()  [unwired: 2 in, 2 out]
          }
          frame Default {
          }
        }
      }
      event "printer_send_template": Value Change {
        n186 = event-data() -> ()  [unwired: 1 in, 6 out]
        n187 = Unbundle By Name(w345) -> ("queue_refnums.PRINTER_queue"=w342:refnum<queue>)
        n188 = To Variant(anything="^XA^CWZ,E:TT0003M_.FNT^FS^XZ\n^XA\n^DFE:A603.ZPL^FS\n^CI33\n\n^FX Field 1 PACKAGING LIST\n\n^FO100,20^CI28^AZN,48,65^FN1^FS\n\n^FX Field 2 Name of manufacture and trademark\n^FO30,150^AZN,20,10^FN2^FS\n^FO40,170^AZN,20,10^FN3^FS\n^FO40,190^^AZN,25,10^FN4^FS\n\n^FX Field 3 Batch/packaging date\n^FO280,95^AZN,28,35^FN5^FS\n^FO330,140^A1,56,30^FN6^FS\n\n^FX Field 4 Quantity box\n^FO810,95^AZN,28,30^FN7^FS\n^FO830,140^A1,56,30^FN8^FS\n\n^FX Field 5 Part number\n^FO15,230^AZN,28,30^FN9^FS\n^FO30,275^A1,56,25^FN10^FS\n\n^FX Field 6 Part name\n^FO15,350^AZN,28,30^FN11^FS\n^FO30,420^AZN,40,45^FN12^FS\n\n^FX Field 7 PSW No.\n^FO15,500^AZN,28,35^FN13^FS\n^FO30,550^AZN,28,35^FN14^FS\n\n^FX Field 8 Batch No.\n^FO500,500^AZN,28,35^FN15^FS\n^FO515,550^A1,56,35^FN16^FS\n\n^FX Field 9 AUSS, TS\n^FO15,635^AZN,28,35^FN17^FS\n^FO30,685^AZN,28,35^FN18^FS\n\n^FX Field 10 Packager\n^FO500,635^AZN,28,35^FN19^FS\n^FO515,685^AZN,28,35^FN20^FS\n\n^FX Field 11 Barcode\n^FO250,755^BY3\n^BCN,80,Y,N,N^FN21^FS\n\n^FX Field 12 Certificate included\n^FO120,910^AZN,48,70^FN22^FS\n\n^FX Lines\n^FO0,72^GB960,1,2^FS\n^FO200,72^GB2,144^FS\n^FO720,72^GB2,144^FS\n^FO0,216^GB960,1,2^FS\n^FO0,336^GB960,1,2^FS\n^FO0,480^GB960,1,2^FS\n^FO0,624^GB960,1,2^FS\n^FO480,480^GB2,264^FS\n^FO0,744^GB960,1,2^FS\n^FO0,888^GB960,1,2^FS\n\n^XZ") -> (Variant=w339:variant)
        n189 = Bundle By Name(cluster=T23 {"state"=enum."send", "variable"=variant} ("element"), "variable"=w339) -> (w340:T23)
        n190 = Enqueue Element(queue=w342, element=w340, error in (no error)=w344) -> (error out=w343:errorcluster)  [unwired: 1 in, 2 out]
      }
      event "printer_send_label": Value Change {
        n191 = event-data() -> ()  [unwired: 1 in, 6 out]
        n192 = Unbundle By Name(w353) -> ("queue_refnums.PRINTER_queue"=w350:refnum<queue>)
        n193 = To Variant(anything="^XA\n^XFE:A603.ZPL^FS\n^CI33\n^FX Field 1 PACKAGING LIST\n\n^FN1^FDУПАКОВОЧНЫИ ЯРЛЫК^FS\n\n^FX Field 2 Name of manufacture and trademark\n^FN2^FDОбщество с ограничонной ^FS\n^FN3^FDотвотстввнностыо ^FS\n^FN4^FD\"РУЛЕВЫЕ СИСТЕМЫ\" ^FS\n\n^FX Field 3 Batch/packaging date\n^FN5^FDДата партии/упаковки^FS\n^FN6^FD24.08.2021^FS\n\n^FX Field 4 Quantity box\n^FN7^FDКол^FS\n^FN8^FD2^FS\n\n^FX Field 5 Part number\n^FN9^FDОбозначение изделия^FS\n^FN10^FD8450022771 (21302-3400012)^FS\n\n^FX Field 6 Part name\n^FN11^FDНаименование изделия:^FS\n^FN12^FDМеханизм рулевой с ^FS\n^FN13^FDуплотнитедем в сборе ^FS\n\n^FX Field 7 PSW No.\n^FN14^FDЗаключение на поставку^FS\n^FN15^FD№:^FS\n\n^FX Field 8 Batch No.\n^FN16^FD№ партии:^FS\n^FN17^FD2370A345^FS\n\n^FX Field 9 AUSS, TS\n^FN18^FDГОСТ, ТУ:^FS\n^FN19^FDеуые1234^FS\n\n^FX Field 10 Packager\n^FN20^FDУпаковщик^FS\n^FN21^FDеуые1234^FS\n\n^FX Field 11 Barcode\n^FO250,755^BY3\n^FN22^FD2370A345001^FS\n\n^FX Field 12 Certificate included\n^FN23^FDСЕРТИФИКАТ ЗДЕСЬ^FS\n\n^XZ" ("String")) -> (Variant=w347:variant)
        n194 = Bundle By Name(cluster=T23 {"state"=enum."send", "variable"=variant} ("element"), "variable"=w347) -> (w348:T23)
        n195 = Enqueue Element(queue=w350, element=w348, error in (no error)=w352) -> (error out=w351:errorcluster)  [unwired: 1 in, 2 out]
      }
      event "print_label_test": Value Change {
        n196 = event-data() -> ()  [unwired: 1 in, 6 out]
        n197 = Unbundle By Name(w356) -> ("queue_refnums.MAIN_queue"=w355:refnum<queue>)
        n198 = Enqueue Element(queue=w355, element=T6 {"state"=enum."print_label", "variable"=variant}, error in (no error)=w358) -> (error out=w357:errorcluster)  [unwired: 1 in, 2 out]
      }
      event Panel Close? {
        n199 = event-data() -> ()  [unwired: 1 in, 4 out]
        n200 = property on="STOP" class="Bool (strict)"("Val(Sgnl)"=TRUE ("Value (Signaling)")) -> ()  [unwired: 2 in, 2 out]
        n201 = event-data("Discard?"=TRUE) -> ()  [unwired: 1 in, 1 out]
      }
      event Timeout {
        n202 = event-data() -> ()  [unwired: 1 in, 3 out]
        n203 = Unbundle By Name(w363) -> ("queue_refnums.MAIN_queue"=w362:refnum<queue>)
        n204 = local read "current_access_level"() -> (w364:i32)
        n205 = case shown="Default" w364 {
          tunnel: w366 -> [w367 w371]
          tunnel: [w367 w375] -> w365
          tunnel: w362 -> [_ w369]
          frame 0 {
          }
          frame Default {
            n206 = Enqueue Element(queue=w369, element=T6 {"state"=enum."USER_logout", "variable"=variant}, error in (no error)=w371) -> (error out=w370:errorcluster)  [unwired: 1 in, 2 out]
            n207 = call "message_popup.vi"("Warning(T)/Info(F)"=TRUE, "error_in"=w370, "Message"="Automatic user logout was performed due to inactivity", "Title"="Automatic Logout", "Button Label"="OK") -> ("error_out"=w375:errorcluster)  [unwired: 6 in]
          }
        }
      }
    }
  }
  n208 = while {
    tunnel: w29 -> [w382]
    shift-right: [w383] -> _
    shift-left: DOCK_MAIN_sequence_state."initialize" ("REWORK_MAIN_sequence_state") -> [w384]
    shift-right: [w381] -> _
    shift-left: _ -> [w380]
    shift-right: [w385] -> w71
    shift-left: w59 -> [w386]
    shift-right: [w377] -> _
    shift-left: T6[] [] -> [w378]
    stop <- w379 stop-if-true
    # "MAIN"
    n209 = case shown="\"preread_gear_data_check\"" w384 {
      tunnel: w386 -> [w397 w408 w435 w479 w496 w522 w534 w556 w571 w596 w646 w665 w692 w717 w769 w776 w802 w823 w833 w858]
      tunnel: [w400 w410 w434 w475 w500 w523 w536 w559 w575 w599 w650 w668 w710 w738 w773 w790 w805 w826 w835 w858] -> w385
      tunnel: [w398 w409 w431 w476 w501 w524 w537 w558 w574 w598 w649 w667 w711 w739 w774 w789 w804 w825 w834 DOCK_MAIN_sequence_state."stop" ("ST_TCP_sequence_state")] -> w383
      tunnel: w382 -> [_ w407 w433 _ w498 _ w532 _ _ _ _ _ _ _ _ _ w800 _ w829 _]
      tunnel: [_ w405 _ _ _ _ _ _ _ _ _ w664 _ _ _ _ _ _ _ _] -> w381
      tunnel: w380 -> [_ _ w432 _ _ _ _ _ w570 _ _ w664 w691 _ w752 _ _ w822 _ _]
      tunnel: [_ _ _ _ _ _ _ _ _ _ _ _ _ _ _ _ _ _ _ TRUE] -> w379
      tunnel: w378 -> [w389 w402 w429 w474 w480 w506 w531 w540 w572 w595 w645 w666 w686 w721 w746 w779 w803 w824 _ w855]
      tunnel: [w389 w401 w429 w474 w480 w506 w531 w540 w572 w595 w645 w666 w685 w721 w745 w779 w803 w824 T6[] [] ("enqueued_states_out") w855] -> w377
      frame "initialize" {
        w392 = ""
        n210 = call "FGV_DOCK_SQL_connection.vi"("options"=FGV_DOCK_SQL_connection."connect", "error_in"=w397) -> ("error_out"=w391:errorcluster)  [unwired: 5 in, 4 out]
        n211 = Unbundle By Name(w391) -> ("status"=w395:bool)
        n212 = local write "SQL_connection_indicator_global"(w395) -> ()
        n213 = call-poly "Get Localized Phrase Compact Interface.vi"("Key"=string[] ["START NEW BATCH"] ("Strings [4]")) -> ("Translated Phrase"=w387:string[])
        n214 = local write "batch_active?"(FALSE ("batch_active?")) -> ()
        n215 = local write "gear_serial_display"(w392) -> ()
        n216 = local write "batch_code_display"(w392) -> ()
        n217 = local write "current_batch_count"(u16 0 ("current_batch_count")) -> ()
        n218 = property on="DOCK_read_gear_data" class="Bool"("DisabledEnum"=T30."Disabled and Grayed Out" ("Disabled")) -> ()  [unwired: 2 in, 2 out]
        n219 = property on="DOCK_start_finish_batch" class="Bool"("Strings [4]"=w387) -> ()  [unwired: 2 in, 2 out]
        n220 = call "DOCK_MAIN_check_for_error.vi"("MAIN_loop_state_in"=DOCK_MAIN_sequence_state."get_next_state", "error_in"=w391) -> ("MAIN_loop_state_out"=w398:T7, "error_out"=w400:errorcluster)  [unwired: 8 in]
      }
      frame "get_next_state" {
        n221 = Empty Array?(array=w402) -> (empty?=w403:bool)
        n222 = case shown="False" w403 {
          tunnel: w408 -> [w416 w426]
          tunnel: w407 -> [_ w425]
          tunnel: [w412 w424] -> w406
          tunnel: [w411 w423] -> w405
          tunnel: [w416 w422] -> w404
          tunnel: w402 -> [w415 w421]
          tunnel: [w414 w421] -> w401
          frame False {
            # "If state is enqueued, proceed with that state"
            n223 = Delete From Array(array=w415, length=1, index=0) -> (deleted portion=w418:T6[], array with subset deleted=w414:T6[])
            n224 = Index Array(array=w418, index=0) -> (element=w413:T6)
            n225 = Unbundle By Name(w413) -> ("variable"=w411:variant, "state"=w412:T7)
          }
          frame True {
            # "If no state enqueued, proceed with queue"
            n226 = Unbundle By Name(w425) -> ("queue_refnums.MAIN_queue"=w427:refnum<queue>)
            n227 = Dequeue Element(queue=w427, error in (no error)=w426) -> (element=w428:T6, error out=w422:errorcluster)  [unwired: 1 in, 2 out]
            n228 = Unbundle By Name(w428) -> ("variable"=w423:variant, "state"=w424:T7)
          }
        }
        n229 = call "DOCK_MAIN_check_for_error.vi"("MAIN_loop_state_in"=w406, "error_in"=w404) -> ("MAIN_loop_state_out"=w409:T7, "error_out"=w410:errorcluster)  [unwired: 8 in]
      }
      frame "USER_login" {
        n230 = Variant To Data(error in=w435, type="", Variant=w432) -> (data=w441:string, error out=w450:errorcluster)
        n231 = Unbundle By Name(w433) -> ("main_ini_file.User table"=w446:string)
        n232 = call "Hash String with SHA-256.vi"("error_n"=w450, "string"=w441) -> ("error_out"=w447:errorcluster, "hash"=w440:string)  [unwired: 8 in]
        n233 = Format Into String(format string="select ID, USER_NAME, PROXY_APP\nfrom %s\nwhere BARCODE_HASH = '%s'\norder by ID desc", w446, w440) -> (resulting string=w449:string)  [unwired: 2 in, 1 out]
        n234 = call "FGV_DOCK_SQL_connection.vi"("options"=FGV_DOCK_SQL_connection."SELECT", "error_in"=w447, "SQL_statement"=w449) -> ("error_out"=w448:errorcluster, "SQL_result"=w445:variant)  [unwired: 4 in, 3 out]
        n235 = Variant To Data(error in=w448, type=string[][] [], Variant=w445) -> (data=w443:string[][], error out=w444:errorcluster)
        n236 = Empty Array?(array=w443) -> (empty?=w442:bool)
        n237 = case shown="True" w442 {
          tunnel: [w462 w470] -> w451
          tunnel: w444 -> [w460 w471]
          tunnel: w443 -> [w457 _]
          tunnel: w441 -> [_ w466]
          tunnel: w440 -> [_ w465]
          frame False {
            w455 = 0 ("index (row)")
            n238 = Index Array(array=w457, index (row) #2=w455, index (col) #2=w455, index (row) #3=w455, index (col) #3=1 ("disabled index (col)"), index (row) #4=w455, index (col) #4=2 ("disabled index (col)")) -> (element #2=w459:string, element #3=w452:string, element #4=w453:string)  [unwired: 2 in, 1 out]
            n239 = Decimal String To Number(string=w453) -> (number=w456:i32)  [unwired: 2 in, 1 out]
            n240 = call "FGV_DOCK_login.vi"("options"=FGV_DOCK_login."login", "error_in"=w460, "access_level_in"=w456, "username_in"=w452, "ID_in"=w459) -> ("error_out"=w462:errorcluster)  [unwired: 2 in, 4 out]
          }
          frame True {
            n241 = call-poly "Get Localized Phrase Compact Interface.vi"("Key"="Scanned card not in database!\nCard: %s\nHash: %s" ("Message")) -> ("Translated Phrase"=w463:string)
            n242 = Format Into String(format string=w463, w466, w465) -> (resulting string=w464:string)  [unwired: 2 in, 1 out]
            n243 = call "message_popup.vi"("Warning(T)/Info(F)"=TRUE, "error_in"=w471, "Message"=w464, "Title"="Login", "Button Label"="OK") -> ("error_out"=w470:errorcluster)  [unwired: 6 in]
          }
        }
        n244 = call "DOCK_MAIN_check_for_error.vi"("MAIN_loop_state_in"=DOCK_MAIN_sequence_state."get_next_state", "error_in"=w451) -> ("MAIN_loop_state_out"=w431:T7, "error_out"=w434:errorcluster)  [unwired: 8 in]
      }
      frame "USER_logout" {
        n245 = call "FGV_DOCK_login.vi"("options"=FGV_DOCK_login."logout", "error_in"=w479) -> ("error_out"=w473:errorcluster)  [unwired: 5 in, 4 out]
        n246 = call "DOCK_MAIN_check_for_error.vi"("MAIN_loop_state_in"=DOCK_MAIN_sequence_state."get_next_state", "error_in"=w473) -> ("MAIN_loop_state_out"=w476:T7, "error_out"=w475:errorcluster)  [unwired: 8 in]
      }
      frame "read_reference_list" {
        n247 = Unbundle By Name(w498) -> ("main_ini_file.Reference table"=w497:string)
        n248 = Format Into String(format string="SELECT DISTINCT REFERENCE_NAME FROM %s\nWHERE NOT REFERENCE_NAME = 'ALL' AND STATION_NMB = 130 ORDER BY REFERENCE_NAME ASC", w497) -> (resulting string=w495:string)  [unwired: 2 in, 1 out]
        n249 = call "FGV_DOCK_SQL_connection.vi"("options"=FGV_DOCK_SQL_connection."EXEC", "error_in"=w496, "SQL_statement"=w495) -> ("error_out"=w486:errorcluster, "SQL_result"=w483:variant, "executed_SQL_statement"=w491:string)  [unwired: 4 in, 2 out]
        n250 = Variant To Data(error in=w486, type=string[][] [], Variant=w483) -> (data=w488:string[][], error out=w485:errorcluster)
        n251 = Index Array(array=w488, index (col)=0 ("disabled index (col)")) -> (element=w484:string[])  [unwired: 1 in]
        n252 = property on="REFERENCE_selector" class="Ring (strict)"("Strings []"=w484) -> (error out=w481:errorcluster)  [unwired: 2 in, 1 out]
        n253 = local read "REFERENCE_selector"() -> (w482:u16)
        n254 = property on="REFERENCE_selector" class="Ring (strict)"(error in=w481, "Val(Sgnl)"=w482) -> ()  [unwired: 1 in, 2 out]
        n255 = call "FGV_DOCK_status_display.vi"("options"=FGV_DOCK_status_display."display", "error_in"=w485, "SQL_statement"=w491, "display_source"="READ REFERENCE LIST") -> ("error_out"=w492:errorcluster)  [unwired: 7 in]
        n256 = call "DOCK_MAIN_check_for_error.vi"("MAIN_loop_state_in"=DOCK_MAIN_sequence_state."get_next_state", "error_in"=w492) -> ("MAIN_loop_state_out"=w501:T7, "error_out"=w500:errorcluster)  [unwired: 8 in]
      }
      frame "read_batch_size_list" {
        n257 = call "FGV_DOCK_SQL_connection.vi"("options"=FGV_DOCK_SQL_connection."EXEC", "error_in"=w522, "SQL_statement"="SELECT DISTINCT BATCH_SIZE FROM DOCK_AUDIT_BATCH_SIZE ORDER BY BATCH_SIZE DESC" ("format string")) -> ("error_out"=w513:errorcluster, "SQL_result"=w511:variant, "executed_SQL_statement"=w518:string)  [unwired: 4 in, 2 out]
        n258 = Variant To Data(error in=w513, type=string[][] [], Variant=w511) -> (data=w515:string[][], error out=w512:errorcluster)
        n259 = Index Array(array=w515, index (col)=0 ("disabled index (col)")) -> (element=w507:string[])  [unwired: 1 in]
        n260 = for {
          tunnel: w507 -> [w528] mode=indexing
          tunnel: [w529] -> w509 mode=indexing
          tunnel: [w526] -> w505 mode=indexing
          n261 = Decimal String To Number(string=w528, default (0L)=u16 0 ("default (0 I32)")) -> (number=w526:u16)  [unwired: 1 in, 1 out]
          n262 = Bundle By Name(cluster=cluster{"String":string, "Value":u16} {"String"="", "Value"=0}, "String"=w528, "Value"=w526) -> (w529:cluster{"String":string, "Value":u16})
        }
        n263 = property on="BATCH_SIZE_selector" class="Ring (strict)"("StringsAndValues[]"=w509) -> (error out=w508:errorcluster)  [unwired: 2 in, 1 out]
        n264 = Index Array(array=w505, index=0) -> (element=w503:u16)
        n265 = property on="BATCH_SIZE_selector" class="Ring (strict)"(error in=w508, "Value"=w503) -> ()  [unwired: 1 in, 2 out]
        n266 = call "FGV_DOCK_status_display.vi"("options"=FGV_DOCK_status_display."display", "error_in"=w512, "SQL_statement"=w518, "display_source"="READ BATCH SIZE LIST") -> ("error_out"=w519:errorcluster)  [unwired: 7 in]
        n267 = call "DOCK_MAIN_check_for_error.vi"("MAIN_loop_state_in"=DOCK_MAIN_sequence_state."get_next_state", "error_in"=w519) -> ("MAIN_loop_state_out"=w524:T7, "error_out"=w523:errorcluster)  [unwired: 8 in]
      }
      frame "change_reference" {
        n268 = property on="REFERENCE_selector" class="Ring (strict)"() -> ("RingText.Text"=w535:string)  [unwired: 2 in, 2 out]
        n269 = call "get_reference_data.vi"("active_reference_name"=w535, "error_in"=w534, "all_config_info"=w532) -> ("error_out"=w533:errorcluster)  [unwired: 8 in]
        n270 = call "DOCK_MAIN_check_for_error.vi"("MAIN_loop_state_in"=DOCK_MAIN_sequence_state."get_next_state", "error_in"=w533) -> ("MAIN_loop_state_out"=w537:T7, "error_out"=w536:errorcluster)  [unwired: 8 in]
      }
      frame "start_batch" {
        n271 = property on="REFERENCE_selector" class="Ring (strict)"() -> ("RingText.Text"=w546:string)  [unwired: 2 in, 2 out]
        n272 = local read "BATCH_SIZE_selector"() -> (w539:u16)
        n273 = Format Into String(format string="EXEC DockAuditCreateBatch @ReferenceName = '%s', @DeclaredSize = %d" ("SQL_statement"), w546, w539) -> (resulting string=w547:string)  [unwired: 2 in, 1 out]
        n274 = call "FGV_DOCK_SQL_connection.vi"("options"=FGV_DOCK_SQL_connection."EXEC", "error_in"=w556, "SQL_statement"=w547) -> ("error_out"=w554:errorcluster, "SQL_result"=w553:variant, "executed_SQL_statement"=w549:string)  [unwired: 4 in, 2 out]
        n275 = call "parse_create_batch_response.vi"("error_in"=w554, "SQL_result"=w553) -> ("error_out"=w545:errorcluster, "batch_ID"=w543:string, "batch_code"=w541:string)  [unwired: 7 in]
        n276 = call "FGV_DOCK_batch_ID_buffer.vi"("options"=FGV_DOCK_batch_ID_buffer."buffer_batch_ID", "error_in"=w545, "BATCH_ID"=w543, "BATCH_CODE"=w541) -> ("error_out"=w544:errorcluster)  [unwired: 5 in, 2 out]
        n277 = local write "batch_code_display"(w541) -> ()
        n278 = call "FGV_DOCK_status_display.vi"("options"=FGV_DOCK_status_display."display", "error_in"=w544, "SQL_statement"=w549, "display_source"="START BATCH") -> ("error_out"=w550:errorcluster)  [unwired: 7 in]
        n279 = case shown="No Error" w550 {
          frame No Error {
            w564 = TRUE ("batch_active?")
            n280 = call "FGV_DOCK_multistate_indicator.vi"("options"=FGV_DOCK_multistate_indicator."start_batch") -> ()  [unwired: 10 in, 1 out]
            n281 = local write "current_batch_count"(u16 0 ("current_batch_count")) -> ()
            n282 = call-poly "Get Localized Phrase Compact Interface.vi"("Key"=string[] ["FINISH CURRENT BATCH"] ("Strings [4]")) -> ("Translated Phrase"=w560:string[])
            n283 = local write "batch_active?"(w564) -> ()
            n284 = To Variant(anything=w564) -> (Variant=w565:variant)
            n285 = property on="DOCK_start_finish_batch" class="Bool"("Strings [4]"=w560) -> ()  [unwired: 2 in, 2 out]
            n286 = property on="DOCK_read_gear_data" class="Bool"("DisabledEnum"=T30."Enabled" ("Disabled")) -> ()  [unwired: 2 in, 2 out]
            n287 = call "FGV_DOCK_controls_state.vi"("options"=FGV_DOCK_controls_state."batch_event", "input"=w565) -> ()  [unwired: 8 in, 2 out]
          }
          frame Error {
          }
        }
        n288 = call "DOCK_MAIN_check_for_error.vi"("MAIN_loop_state_in"=DOCK_MAIN_sequence_state."get_next_state", "error_in"=w550) -> ("MAIN_loop_state_out"=w558:T7, "error_out"=w559:errorcluster)  [unwired: 8 in]
      }
      frame "reload_batch" {
        n289 = call "DOCK_MAIN_get_reload_data.vi"("error_in"=w571, "variable"=w570) -> ("error_out"=w568:errorcluster, "reload_data"=w569:T25)  [unwired: 8 in]
        n290 = case shown="No Error" w568 {
          tunnel: w569 -> [w587 _]
          frame No Error {
            w577 = TRUE ("batch_active?")
            n291 = Unbundle By Name(w587) -> ("part_number"=w583:string, "declared_size"=w584:u16, "batch_code"=w586:string, "current_size"=w585:u16)
            n292 = local write "reload_batch_size"(w584) -> ()
            n293 = local write "batch_code_display"(w586) -> ()
            n294 = local write "reload_part_number"(w583) -> ()
            n295 = call "FGV_DOCK_multistate_indicator.vi"("options"=FGV_DOCK_multistate_indicator."start_batch") -> ()  [unwired: 10 in, 1 out]
            n296 = local write "current_batch_count"(w585) -> ()
            n297 = call-poly "Get Localized Phrase Compact Interface.vi"("Key"=string[] ["FINISH CURRENT BATCH"] ("Strings [4]")) -> ("Translated Phrase"=w576:string[])
            n298 = local write "batch_active?"(w577) -> ()
            n299 = To Variant(anything=w577) -> (Variant=w580:variant)
            n300 = local write "reload_active?"(w577) -> ()
            n301 = property on="DOCK_start_finish_batch" class="Bool"("Strings [4]"=w576) -> ()  [unwired: 2 in, 2 out]
            n302 = property on="DOCK_read_gear_data" class="Bool"("DisabledEnum"=T30."Enabled" ("Disabled")) -> ()  [unwired: 2 in, 2 out]
            n303 = call "FGV_DOCK_controls_state.vi"("options"=FGV_DOCK_controls_state."reload_event", "input"=w580) -> ()  [unwired: 8 in, 2 out]
          }
          frame Error {
          }
        }
        n304 = call "DOCK_MAIN_check_for_error.vi"("MAIN_loop_state_in"=DOCK_MAIN_sequence_state."get_next_state", "error_in"=w568) -> ("MAIN_loop_state_out"=w574:T7, "error_out"=w575:errorcluster)  [unwired: 8 in]
      }
      frame "finish_batch?" {
        n305 = local read "reload_batch_size"() -> (w591:u16)
        n306 = local read "BATCH_SIZE_selector"() -> (w590:u16)
        n307 = local read "reload_active?"() -> (w592:bool)
        n308 = local read "current_batch_count"() -> (w593:u16)
        n309 = Select(t=w591, s=w592, f=w590) -> (s? t:f=w589:u16)
        n310 = Greater Or Equal?(x=w593, y=w589) -> (x >= y?=w594:bool)
        n311 = case shown="True" w594 {
          tunnel: [w601 w603] -> w597
          tunnel: w596 -> [w601 w616]
          tunnel: w593 -> [_ w605]
          tunnel: [DOCK_MAIN_sequence_state."get_next_state" ("MAIN_loop_state_in") w602] -> w588
          frame False {
          }
          frame True {
            n312 = local read "batch_code_display"() -> (w614:string)
            n313 = call "FGV_DOCK_batch_ID_buffer.vi"("options"=FGV_DOCK_batch_ID_buffer."get_ID_for_batch", "error_in"=w616, "BATCH_CODE"=w614) -> ("error_out"=w610:errorcluster, "ID_out"=w612:string)  [unwired: 6 in, 1 out]
            n314 = Format Into String(format string="EXEC DockAuditFinishBatch @BatchID = %s, @ActualSize = %d", w612, w605) -> (resulting string=w609:string)  [unwired: 2 in, 1 out]
            n315 = call "FGV_DOCK_SQL_connection.vi"("options"=FGV_DOCK_SQL_connection."EXEC", "error_in"=w610, "SQL_statement"=w609) -> ("error_out"=w607:errorcluster, "SQL_result"=w606:variant, "executed_SQL_statement"=w608:string)  [unwired: 4 in, 2 out]
            n316 = call "parse_finish_batch_response.vi"("error_in"=w607, "SQL_result"=w606) -> ("error_out"=w604:errorcluster)  [unwired: 9 in]
            n317 = case shown="No Error" w604 {
              tunnel: [DOCK_MAIN_sequence_state."print_label" ("MAIN_loop_state_in") DOCK_MAIN_sequence_state."error" ("MAIN_loop_state_in")] -> w602
              frame No Error {
                w624 = FALSE ("batch_active?")
                n318 = property on="DOCK_read_gear_data" class="Bool"("DisabledEnum"=T30."Disabled and Grayed Out" ("Disabled")) -> ()  [unwired: 2 in, 2 out]
                n319 = call "message_popup.vi"("Message"="Closing current batch because it's full. Start new batch to continue packaging.", "Title"="BATCH FULL", "Button Label"="OK") -> ()  [unwired: 8 in, 1 out]
                n320 = call-poly "Get Localized Phrase Compact Interface.vi"("Key"=string[] ["START NEW BATCH"] ("Strings [4]")) -> ("Translated Phrase"=w619:string[])
                n321 = property on="DOCK_start_finish_batch" class="Bool"("Strings [4]"=w619) -> ()  [unwired: 2 in, 2 out]
                n322 = To Variant(anything=w624) -> (Variant=w627:variant)
                n323 = local write "batch_active?"(w624) -> ()
                n324 = local write "reload_active?"(w624) -> ()
                n325 = call "FGV_DOCK_controls_state.vi"("options"=FGV_DOCK_controls_state."batch_event", "input"=w627) -> ()  [unwired: 8 in, 2 out]
                n326 = call "FGV_DOCK_multistate_indicator.vi"("options"=FGV_DOCK_multistate_indicator."finish_batch") -> ()  [unwired: 10 in, 1 out]
              }
              frame Error {
              }
            }
            n327 = call "FGV_DOCK_status_display.vi"("options"=FGV_DOCK_status_display."display", "error_in"=w604, "SQL_statement"=w608, "display_source"="FINISH BATCH") -> ("error_out"=w603:errorcluster)  [unwired: 7 in]
          }
        }
        n328 = call "DOCK_MAIN_check_for_error.vi"("MAIN_loop_state_in"=w588, "error_in"=w597) -> ("MAIN_loop_state_out"=w598:T7, "error_out"=w599:errorcluster)  [unwired: 8 in]
      }
      frame "finish_batch" {
        n329 = local read "current_batch_count"() -> (w644:u16)
        n330 = local read "batch_code_display"() -> (w640:string)
        n331 = call "FGV_DOCK_batch_ID_buffer.vi"("options"=FGV_DOCK_batch_ID_buffer."get_ID_for_batch", "error_in"=w646, "BATCH_CODE"=w640) -> ("error_out"=w636:errorcluster, "ID_out"=w638:string)  [unwired: 6 in, 1 out]
        n332 = Format Into String(format string="EXEC DockAuditFinishBatch @BatchID = %s, @ActualSize = %d", w638, w644) -> (resulting string=w635:string)  [unwired: 2 in, 1 out]
        n333 = call "FGV_DOCK_SQL_connection.vi"("options"=FGV_DOCK_SQL_connection."EXEC", "error_in"=w636, "SQL_statement"=w635) -> ("error_out"=w633:errorcluster, "SQL_result"=w631:variant, "executed_SQL_statement"=w634:string)  [unwired: 4 in, 2 out]
        n334 = call "parse_finish_batch_response.vi"("error_in"=w633, "SQL_result"=w631) -> ("error_out"=w632:errorcluster)  [unwired: 9 in]
        n335 = case shown="No Error" w632 {
          frame No Error {
            w652 = FALSE ("batch_active?")
            n336 = property on="DOCK_read_gear_data" class="Bool"("DisabledEnum"=T30."Disabled and Grayed Out" ("Disabled")) -> ()  [unwired: 2 in, 2 out]
            n337 = call-poly "Get Localized Phrase Compact Interface.vi"("Key"=string[] ["START NEW BATCH"] ("Strings [4]")) -> ("Translated Phrase"=w651:string[])
            n338 = property on="DOCK_start_finish_batch" class="Bool"("Strings [4]"=w651) -> ()  [unwired: 2 in, 2 out]
            n339 = To Variant(anything=w652) -> (Variant=w655:variant)
            n340 = local write "batch_active?"(w652) -> ()
            n341 = local write "reload_active?"(w652) -> ()
            n342 = call "FGV_DOCK_controls_state.vi"("options"=FGV_DOCK_controls_state."batch_event", "input"=w655) -> ()  [unwired: 8 in, 2 out]
            n343 = call "FGV_DOCK_multistate_indicator.vi"("options"=FGV_DOCK_multistate_indicator."finish_batch") -> ()  [unwired: 10 in, 1 out]
          }
          frame Error {
          }
        }
        n344 = call "FGV_DOCK_status_display.vi"("options"=FGV_DOCK_status_display."display", "error_in"=w632, "SQL_statement"=w634, "display_source"="FINISH BATCH") -> ("error_out"=w647:errorcluster)  [unwired: 7 in]
        n345 = call "DOCK_MAIN_check_for_error.vi"("MAIN_loop_state_in"=DOCK_MAIN_sequence_state."print_label", "error_in"=w647) -> ("MAIN_loop_state_out"=w649:T7, "error_out"=w650:errorcluster)  [unwired: 8 in]
      }
      frame "preread_gear_data_check" {
        n346 = call "FGV_DOCK_controls_state.vi"("options"=FGV_DOCK_controls_state."get_gear_loaded_status") -> ("error_out"=w661:errorcluster, "output"=w662:variant)  [unwired: 9 in]
        n347 = Variant To Data(error in=w661, type=TRUE, Variant=w662) -> (data=w658:bool)  [unwired: 1 out]
        n348 = case shown="True" w658 {
          tunnel: [DOCK_MAIN_sequence_state."read_gear_data" ("MAIN_loop_state_in") w675] -> w663
          frame False {
          }
          frame True {
            n349 = call "confirm_popup_dock_audit.vi"("Warning(T)/Inf(F)"=TRUE, "Title"="CURRENT GEAR NOT FINISHED", "True Label"="OK", "Message"="Current gear is not finished. Are you sure you want to load new gear?") -> ("Result"=w670:bool)  [unwired: 6 in, 1 out]
            n350 = case shown="True" w670 {
              tunnel: [DOCK_MAIN_sequence_state."get_next_state" ("MAIN_loop_state_in") DOCK_MAIN_sequence_state."read_gear_data" ("MAIN_loop_state_in")] -> w675
              frame False {
              }
              frame True {
              }
            }
          }
        }
        n351 = call "DOCK_MAIN_check_for_error.vi"("MAIN_loop_state_in"=w663, "error_in"=w665) -> ("MAIN_loop_state_out"=w667:T7, "error_out"=w668:errorcluster)  [unwired: 8 in]
      }
      frame "read_gear_data" {
        n352 = local read "reload_active?"() -> (w680:bool)
        n353 = local read "reload_part_number"() -> (w679:string)
        n354 = call "check_part_number_ref.vi"("reload_part_number"=w679, "reload_active?"=w680, "error_in"=w692, "variable"=w691) -> ("error_out"=w690:errorcluster, "reload_part_number"=w678:string, "gear_serial"=w681:string, "part_number_ref_status"=w687:string)  [unwired: 4 in]
        n355 = local write "reload_part_number"(w678) -> ()
        n356 = To Variant(anything=w681) -> (Variant=w708:variant)
        n357 = Format Into String(format string="select top 1 PRODUCTION_PARTS.ID, PRODUCTION_PARTS.CREATION_TIME, PRODUCTION_PARTS.LAST_STATION_NMB, PRODUCTION_PARTS.LAST_STATUS, PRODUCTION_PINIONS.PINION_SERIAL, DOCK_AUDIT_BATCHES.BATCH_CODE, PRODUCTION_PARTS.PINION_ID, PRODUCTION_PARTS.BATCH_ID\nfrom PRODUCTION_PARTS \nleft join PRODUCTION_PINIONS on PRODUCTION_PARTS.PINION_ID = PRODUCTION_PINIONS.ID\nleft join DOCK_AUDIT_BATCHES on PRODUCTION_PARTS.BATCH_ID = DOCK_AUDIT_BATCHES.ID\nwhere PART_SERIAL = '%s'", w681) -> (resulting string=w702:string)  [unwired: 2 in, 1 out]
        n358 = call "FGV_DOCK_records_display.vi"("options"=FGV_DOCK_records_display."set_serial", "input"=w708) -> ()  [unwired: 8 in, 2 out]
        n359 = local write "gear_serial_display"(w681) -> ()
        n360 = call "FGV_DOCK_SQL_connection.vi"("options"=FGV_DOCK_SQL_connection."EXEC", "error_in"=w690, "SQL_statement"=w702) -> ("error_out"=w701:errorcluster, "SQL_result"=w706:variant, "executed_SQL_statement"=w705:string)  [unwired: 4 in, 2 out]
        n361 = call "FGV_DOCK_records_display.vi"("options"=FGV_DOCK_records_display."set_header", "error_in"=w701, "input"=w706) -> ("error_out"=w703:errorcluster)  [unwired: 7 in, 1 out]
        n362 = call "DOCK_GEAR_get_operations_and_results.vi"("executed_SQL_statement_in"=w705, "error_in"=w703, "SQL_result"=w706) -> ("error_out"=w689:errorcluster, "current_batch_ID"=w684:string, "NOK_stations"=w688:string[], "executed_SQL_statement_out"=w704:string)  [unwired: 5 in]
        n363 = local read "current_access_level"() -> (w683:i32)
        n364 = local read "batch_code_display"() -> (w682:string)
        n365 = call "FGV_DOCK_records_display.vi"("options"=FGV_DOCK_records_display."display", "error_in"=w689) -> ("error_out"=w707:errorcluster)  [unwired: 8 in, 1 out]
        n366 = call "evaluate_gear_data_read.vi"("active_batch_code"=w682, "current_access_level"=w683, "current_batch_ID"=w684, "NOK_stations"=w688, "part_number_ref_status"=w687, "enqueued_states_in"=w686) -> ("enqueued_states_out"=w685:T6[])  [unwired: 5 in]
        n367 = call "FGV_DOCK_status_display.vi"("options"=FGV_DOCK_status_display."display", "error_in"=w707, "SQL_statement"=w704, "display_source"="READ GEAR DATA") -> ("error_out"=w693:errorcluster)  [unwired: 7 in]
        n368 = call "DOCK_MAIN_check_for_error.vi"("MAIN_loop_state_in"=DOCK_MAIN_sequence_state."get_next_state", "error_in"=w693) -> ("MAIN_loop_state_out"=w711:T7, "error_out"=w710:errorcluster)  [unwired: 8 in]
      }
      frame "refresh_gear_data" {
        n369 = call "FGV_DOCK_records_display.vi"("options"=FGV_DOCK_records_display."get_serial", "error_in"=w717) -> ("error_out"=w716:errorcluster, "output"=w715:variant)  [unwired: 8 in]
        n370 = Variant To Data(error in=w716, type="", Variant=w715) -> (data=w712:string, error out=w720:errorcluster)
        n371 = To Variant(anything=w712) -> (Variant=w736:variant)
        n372 = Format Into String(format string="select top 1 PRODUCTION_PARTS.ID, PRODUCTION_PARTS.CREATION_TIME, PRODUCTION_PARTS.LAST_STATION_NMB, PRODUCTION_PARTS.LAST_STATUS, PRODUCTION_PINIONS.PINION_SERIAL, DOCK_AUDIT_BATCHES.BATCH_CODE, PRODUCTION_PARTS.PINION_ID, PRODUCTION_PARTS.BATCH_ID\nfrom PRODUCTION_PARTS \nleft join PRODUCTION_PINIONS on PRODUCTION_PARTS.PINION_ID = PRODUCTION_PINIONS.ID\nleft join DOCK_AUDIT_BATCHES on PRODUCTION_PARTS.BATCH_ID = DOCK_AUDIT_BATCHES.ID\nwhere PART_SERIAL = '%s'", w712) -> (resulting string=w730:string)  [unwired: 2 in, 1 out]
        n373 = call "FGV_DOCK_records_display.vi"("options"=FGV_DOCK_records_display."set_serial", "input"=w736) -> ()  [unwired: 8 in, 2 out]
        n374 = local write "gear_serial_display"(w712) -> ()
        n375 = call "FGV_DOCK_SQL_connection.vi"("options"=FGV_DOCK_SQL_connection."EXEC", "error_in"=w720, "SQL_statement"=w730) -> ("error_out"=w729:errorcluster, "SQL_result"=w734:variant, "executed_SQL_statement"=w733:string)  [unwired: 4 in, 2 out]
        n376 = call "FGV_DOCK_records_display.vi"("options"=FGV_DOCK_records_display."set_header", "error_in"=w729, "input"=w734) -> ("error_out"=w731:errorcluster)  [unwired: 7 in, 1 out]
        n377 = call "DOCK_GEAR_get_operations_and_results.vi"("executed_SQL_statement_in"=w733, "error_in"=w731, "SQL_result"=w734) -> ("error_out"=w722:errorcluster, "executed_SQL_statement_out"=w732:string)  [unwired: 5 in, 2 out]
        n378 = call "FGV_DOCK_records_display.vi"("options"=FGV_DOCK_records_display."display", "error_in"=w722) -> ("error_out"=w735:errorcluster)  [unwired: 8 in, 1 out]
        n379 = call "FGV_DOCK_status_display.vi"("options"=FGV_DOCK_status_display."display", "error_in"=w735, "SQL_statement"=w732, "display_source"="REFRESH GEAR DATA") -> ("error_out"=w723:errorcluster)  [unwired: 7 in]
        n380 = call "DOCK_MAIN_check_for_error.vi"("MAIN_loop_state_in"=DOCK_MAIN_sequence_state."get_next_state", "error_in"=w723) -> ("MAIN_loop_state_out"=w739:T7, "error_out"=w738:errorcluster)  [unwired: 8 in]
      }
      frame "save_gear_to_batch" {
        # "refresh gear data\ncall finish_batch? to check if batch full"
        n381 = local read "batch_code_display"() -> (w741:string)
        n382 = Variant To Data(type=0, Variant=w752) -> (data=w742:i32)  [unwired: 1 in, 1 out]
        n383 = call "FGV_DOCK_batch_ID_buffer.vi"("options"=FGV_DOCK_batch_ID_buffer."get_ID_for_batch", "error_in"=w769, "BATCH_CODE"=w741) -> ("error_out"=w766:errorcluster, "ID_out"=w767:string)  [unwired: 6 in, 1 out]
        n384 = call "FGV_DOCK_controls_state.vi"("options"=FGV_DOCK_controls_state."gear_saved_event") -> ()  [unwired: 9 in, 2 out]
        n385 = call "FGV_DOCK_records_display.vi"("options"=FGV_DOCK_records_display."get_gear_ID", "error_in"=w766) -> ("error_out"=w764:errorcluster, "output"=w763:variant)  [unwired: 8 in]
        n386 = Variant To Data(error in=w764, type="", Variant=w763) -> (data=w761:string, error out=w759:errorcluster)
        n387 = call "FGV_DOCK_login.vi"("options"=FGV_DOCK_login."get_login_info", "error_in"=w759) -> ("error_out"=w758:errorcluster, "ID_out"=w760:string)  [unwired: 5 in, 3 out]
        n388 = Format Into String(format string="EXEC DockAuditSaveGearToBatch @IsGearOK = %d, @BatchCode = '%s', @BatchID = '%s', @GearID = %s, @UserID = %s", w742, w741, w767, w761, w760) -> (resulting string=w772:string)  [unwired: 2 in, 1 out]
        n389 = local read "current_batch_count"() -> (w751:u16)
        n390 = call "FGV_DOCK_SQL_connection.vi"("options"=FGV_DOCK_SQL_connection."EXEC", "error_in"=w758, "SQL_statement"=w772) -> ("error_out"=w748:errorcluster, "SQL_result"=w749:variant, "executed_SQL_statement"=w754:string)  [unwired: 4 in, 2 out]
        n391 = call "parse_save_gear_to_batch_response.vi"("gear_ok?"=w742, "error_in"=w748, "SQL_result"=w749, "current_batch_count"=w751) -> ("error_out"=w747:errorcluster, "current_batch_count"=w750:u16)  [unwired: 6 in]
        n392 = local write "current_batch_count"(w750) -> ()
        n393 = call "FGV_DOCK_status_display.vi"("options"=FGV_DOCK_status_display."display", "error_in"=w747, "SQL_statement"=w754, "display_source"="SAVE GEAR TO BATCH") -> ("error_out"=w743:errorcluster)  [unwired: 7 in]
        n394 = Build Array (concatenate)(w746, T6[] [{"state"=enum."refresh_gear_data", "variable"=variant}, {"state"=enum."finish_batch?", "variable"=variant}] ("array")) -> (w745:T6[])
        n395 = call "DOCK_MAIN_check_for_error.vi"("MAIN_loop_state_in"=DOCK_MAIN_sequence_state."get_next_state", "error_in"=w743) -> ("MAIN_loop_state_out"=w774:T7, "error_out"=w773:errorcluster)  [unwired: 8 in]
      }
      frame "clear_gear_data" {
        n396 = call "FGV_DOCK_multistate_indicator.vi"("options"=FGV_DOCK_multistate_indicator."gear_clear", "error_in"=w776) -> ("error_out"=w777:errorcluster)  [unwired: 9 in]
        n397 = call "FGV_DOCK_records_display.vi"("options"=FGV_DOCK_records_display."clear", "error_in"=w777) -> ("error_out"=w786:errorcluster)  [unwired: 8 in, 1 out]
        n398 = local write "gear_serial_display"("") -> ()
        n399 = call "FGV_DOCK_status_display.vi"("options"=FGV_DOCK_status_display."clear", "error_in"=w786) -> ("error_out"=w781:errorcluster)  [unwired: 9 in]
        n400 = To Variant(anything=FALSE) -> (Variant=w783:variant)
        n401 = call "FGV_DOCK_controls_state.vi"("options"=FGV_DOCK_controls_state."gear_event", "error_in"=w781, "input"=w783) -> ("error_out"=w780:errorcluster)  [unwired: 7 in, 1 out]
        n402 = call "DOCK_MAIN_check_for_error.vi"("MAIN_loop_state_in"=DOCK_MAIN_sequence_state."get_next_state", "error_in"=w780) -> ("MAIN_loop_state_out"=w789:T7, "error_out"=w790:errorcluster)  [unwired: 8 in]
      }
      frame "print_label" {
        n403 = local read "current_batch_count"() -> (w795:u16)
        n404 = local read "batch_code_display"() -> (w794:string)
        n405 = local read "current_username"() -> (w793:string)
        n406 = local read "reload_active?"() -> (w796:bool)
        n407 = Number To Decimal String(number=w795) -> (decimal integer string=w797:string)  [unwired: 1 in]
        n408 = call "prepare_label.vi"("error_in"=w802, "reload_active?"=w796) -> ("error_out"=w801:errorcluster, "label_fields"=w799:T29)  [unwired: 8 in]
        n409 = Bundle By Name(cluster=w799, "quantity"=w797, "batch_number"=w794, "barcode"=w794, "packager"=w793) -> (w798:T29)
        n410 = call "print_label.vi"("all_config_info"=w800, "error_in"=w801, "label_fields"=w798) -> ("error_out"=w792:errorcluster)  [unwired: 8 in]
        n411 = flat-sequence {
          tunnel: w792 -> [_]
          frame #0 {
            n412 = local write "current_batch_count"(u16 0 ("current_batch_count")) -> ()
            n413 = local write "batch_code_display"("") -> ()
          }
        }
        n414 = call "DOCK_MAIN_check_for_error.vi"("MAIN_loop_state_in"=DOCK_MAIN_sequence_state."get_next_state", "error_in"=w792) -> ("MAIN_loop_state_out"=w804:T7, "error_out"=w805:errorcluster)  [unwired: 8 in]
      }
      frame "report_get" {
        n415 = Variant To Data(error in=w823, type="", Variant=w822) -> (data=w819:string, error out=w820:errorcluster)
        n416 = call "DOCK_REPORT_CBATCH_get_data_from_SQL.vi"("error_in"=w820, "cbatch_code"=w819) -> ("error_out"=w817:errorcluster, "SQL_result"=w818:variant, "executed_SQL_statement"=w809:string)  [unwired: 7 in]
        n417 = call "FGV_DOCK_REPORT_records_display.vi"("options"=FGV_DOCK_REPORT_records_display."set_records", "error_in"=w817, "input"=w818) -> ("error_out"=w814:errorcluster)  [unwired: 7 in, 1 out]
        n418 = call "FGV_DOCK_REPORT_records_display.vi"("options"=FGV_DOCK_REPORT_records_display."display", "error_in"=w814) -> ("error_out"=w812:errorcluster)  [unwired: 8 in, 1 out]
        n419 = call "FGV_DOCK_REPORT_status_display.vi"("options"=FGV_DOCK_REPORT_status_display."display", "error_in"=w812, "SQL_statement"=w809, "display_source"="DOCK BATCH REPORT") -> ("error_out"=w811:errorcluster)  [unwired: 7 in]
        n420 = call "DOCK_MAIN_check_for_error.vi"("MAIN_loop_state_in"=DOCK_MAIN_sequence_state."get_next_state", "error_in"=w811) -> ("MAIN_loop_state_out"=w825:T7, "error_out"=w826:errorcluster)  [unwired: 8 in]
      }
      frame "error" {
        n421 = call "FGV_DOCK_error_buffer.vi"("thread"=DOCK_thread."MAIN", "option"=FGV_DOCK_error_buffer."display", "error_in"=w833) -> ("error_out"=w832:errorcluster)  [unwired: 7 in, 1 out]
        n422 = call "FGV_DOCK_SQL_connection.vi"("options"=FGV_DOCK_SQL_connection."connection_active?", "error_in"=w832) -> ("error_out"=w838:errorcluster, "connection_active?"=w837:bool)  [unwired: 5 in, 3 out]
        n423 = case shown="False" w837 {
          tunnel: [w844 DOCK_MAIN_sequence_state."get_next_state" ("ST_TCP_sequence_state")] -> w834
          tunnel: [w842 w853] -> w835
          tunnel: w838 -> [w847 w853]
          tunnel: w829 -> [w840 _]
          frame False {
            # "ERROR WITH CONNECTION"
            n424 = Unbundle By Name(w840) -> ("queue_refnums.MAIN_queue"=w839:refnum<queue>)
            n425 = local write "SQL_connection_indicator_global"(TRUE ("SQL_connections_indicator_global")) -> ()
            n426 = call "FGV_DOCK_SQL_connection.vi"("options"=FGV_DOCK_SQL_connection."disconnect", "error_in"=w847) -> ("error_out"=w850:errorcluster)  [unwired: 5 in, 4 out]
            n427 = call <vilib>:"Clear Errors.vi"("error in (no error)"=w850) -> ("error out"=w843:errorcluster)  [unwired: 5 in, 1 out]
            n428 = Preview Queue Element(queue=w839, timeout in ms (-1)=0, error in (no error)=w843) -> (element=w846:T6, error out=w842:errorcluster)  [unwired: 2 out]
            n429 = Unbundle By Name(w846) -> ("state"=w841:T7)
            n430 = case shown="Default" w841 {
              selector: w841 -> [_ w852]
              tunnel: [DOCK_MAIN_sequence_state."initialize" ("ST_TCP_sequence_state") w852] -> w844
              frame Default {
              }
              frame "stop" {
              }
            }
          }
          frame True {
            # "ERROR WITH SQL STATEMENT OR SIMILAR"
          }
        }
        n431 = call "wait_on_initialization.vi"("state"=w834) -> ()  [unwired: 11 in]
      }
      frame "stop" {
      }
    }
  }
  n432 = while {
    tunnel: w29 -> [w865]
    shift-right: [w864] -> _
    shift-left: DOCK_SCANNER_sequence_state."initialize" ("DOCK_SCANNER_sequence_state") -> [w859]
    shift-right: [w862] -> _
    shift-left: "" -> [w860]
    shift-right: [w863] -> _
    shift-left: _ -> [w861]
    shift-right: [w867] -> w70
    shift-left: w59 -> [w868]
    stop <- w866 stop-if-true
    # "SCANNER"
    n433 = case shown="\"read\"" w859 {
      tunnel: w868 -> [w884 w899 w925 w962 w971]
      tunnel: [w887 w897 w928 w954 w969] -> w867
      tunnel: [w885 w893 w926 w953 DOCK_SCANNER_sequence_state."stop" ("state")] -> w864
      tunnel: [_ _ _ _ TRUE] -> w866
      tunnel: w865 -> [w882 w898 w919 w957 _]
      tunnel: [w871 w888 w924 w963 refnum<visa-resource-name> refnum ("VISA resource name out")] -> w863
      tunnel: w861 -> [_ w888 w924 w963 w968]
      tunnel: w860 -> [_ w895 w915 _ _]
      tunnel: ["" w895 w917 "" ""] -> w862
      frame "initialize" {
        n434 = Unbundle By Name(w882) -> ("main_ini_file.SCANNER Termination char"=w872:u8, "main_ini_file.SCANNER COM port"=w881:u16, "main_ini_file.SCANNER Baud rate"=w877:u32, "main_ini_file.SCANNER Data bits"=w876:u16, "main_ini_file.SCANNER Pairity"=w875:enum16{"None", "Odd", "Even", "Mark", "Space"}, "main_ini_file.SCANNER Stop bits"=w874:u16, "main_ini_file.SCANNER Flow control"=w873:u16)
        n435 = Number To Decimal String(number=w881) -> (decimal integer string=w880:string)  [unwired: 1 in]
        n436 = Concatenate Strings("COM" ("string"), w880) -> (w878:string)
        n437 = call-poly "VISA Configure Serial Port"("VISA resource name"=w878, "timeout (10sec)"=u32 150, "termination char\n(0xA = '\\n' = LF)"=w872, "baud rate (9600)"=w877, "data bits (8)"=w876, "parity (0:none)"=w875, "error in (no error)"=w884, "stop bits (10: 1 bit)"=w874, "flow control (0:none)"=w873) -> ("VISA resource name out"=w871:refnum<visa-resource-name>, "error out"=w883:errorcluster)  [unwired: 1 in, 4 out]
        n438 = call "DOCK_SCANNER_check_for_error.vi"("SCANNER_loop_state_in"=DOCK_SCANNER_sequence_state."get_next_state" ("SQL_EDITOR_sequence_state"), "error_in"=w883) -> ("SCANNER_loop_state_out"=w885:T17, "error_out"=w887:errorcluster)  [unwired: 8 in]
      }
      frame "get_next_state" {
        n439 = Unbundle By Name(w898) -> ("queue_refnums.SCANNER_queue"=w900:refnum<queue>)
        n440 = Dequeue Element(queue=w900, timeout in ms (-1)=0, error in (no error)=w899) -> (element=w889:T24, timed out?=w890:bool, error out=w892:errorcluster)  [unwired: 1 out]
        n441 = case shown="False" w890 {
          tunnel: w889 -> [w906 _]
          tunnel: [w902 DOCK_SCANNER_sequence_state."read" ("REWORK_SCANNER_sequence_state")] -> w894
          tunnel: [w901 w914] -> w891
          tunnel: w892 -> [w905 w914]
          tunnel: w888 -> [w903 _]
          frame False {
            # "clear buffers\non read start"
            n442 = Unbundle By Name(w906) -> ("state"=w904:T17)
            n443 = case shown="\"read\"" w904 {
              selector: w904 -> [w908 w909]
              tunnel: w905 -> [w907 w912]
              tunnel: [w907 w911] -> w901
              tunnel: w903 -> [_ w910]
              tunnel: [w908 w909] -> w902
              frame Default {
              }
              frame "read" {
                n444 = VISA Clear(VISA resource name=w910, error in (no error)=w912) -> (error out=w911:errorcluster)  [unwired: 1 out]
              }
            }
          }
          frame True {
          }
        }
        n445 = call "DOCK_SCANNER_check_for_error.vi"("SCANNER_loop_state_in"=w894, "error_in"=w891) -> ("SCANNER_loop_state_out"=w893:T17, "error_out"=w897:errorcluster)  [unwired: 8 in]
      }
      frame "read" {
        # "timeout"
        n446 = VISA Read(VISA resource name=w924, byte count=u32 9999, error in (no error)=w925) -> (read buffer=w918:string, return count=w920:u32, error out=w916:errorcluster)  [unwired: 1 out]
        n447 = case shown="No Error" w916 {
          tunnel: w920 -> [_ w946]
          tunnel: w919 -> [w936 _]
          tunnel: w918 -> [w932 w945]
          tunnel: [w935 w944] -> w917
          tunnel: w915 -> [w933 w943]
          frame No Error {
            # "no (timeout) error means that termination character was encountered"
            n448 = Concatenate Strings(w933, w932) -> (w930:string)
            n449 = call <vilib>:"Trim Whitespace.vi"("string"=w930) -> ("trimmed string"=w929:string)  [unwired: 1 in]
            n450 = Not Equal?(x=w930, y="NoRead\r\n" ("x")) -> (x != y?=w931:bool)
            n451 = case shown="True" w931 {
              tunnel: w936 -> [w939 _]
              tunnel: ["" ""] -> w935
              tunnel: w929 -> [w938 _]
              frame True {
                # "read successful - send data and start new read"
                n452 = local read "batch_active?"() -> (w937:bool)
                n453 = control-ref of="DOCK_gear_serial"() -> (w940:refnum<vi>)
                n454 = call "parse_scanner_data.vi"("batch_active?"=w937, "DOCK_gear_serial"=w940, "SCANNER_data"=w938, "all_config_info"=w939) -> ()  [unwired: 8 in]
              }
              frame False {
                # "read completed, but unsuccessful - clear buffer and start read again"
              }
            }
          }
          frame Error {
            # "(timeout) error and some bytes read means that timeout occured before encountering termination character"
            n455 = case shown="0" w946 {
              tunnel: w945 -> [w948 _]
              tunnel: [w947 w950] -> w944
              tunnel: w943 -> [w949 w950]
              frame Default {
                # "if error and some bytes read, append new bytes (probably timeout, if not error case will take care of it)"
                n456 = Concatenate Strings(w949, w948) -> (w947:string)
              }
              frame 0 {
                # "if error and no bytes read, do nothing (probably timeout, if not error case will take care of it)"
                # "if error and no bytes read, do nothing (probably timeout, if not error case takes care of it"
              }
            }
          }
        }
        n457 = call <vilib>:"Clear Errors.vi"("error in (no error)"=w916, "specific error code to clear (0: all)"=-1073807339) -> ("error out"=w922:errorcluster)  [unwired: 4 in, 1 out]
        n458 = call "DOCK_SCANNER_check_for_error.vi"("SCANNER_loop_state_in"=DOCK_SCANNER_sequence_state."get_next_state" ("state"), "error_in"=w922) -> ("SCANNER_loop_state_out"=w926:T17, "error_out"=w928:errorcluster)  [unwired: 8 in]
      }
      frame "error" {
        n459 = Unbundle By Name(w957) -> ("queue_refnums.SCANNER_queue"=w956:refnum<queue>)
        n460 = call "FGV_DOCK_error_buffer.vi"("thread"=DOCK_thread."SCANNER", "option"=FGV_DOCK_error_buffer."display", "error_in"=w962) -> ("error_out"=w955:errorcluster)  [unwired: 7 in, 1 out]
        n461 = Preview Queue Element(queue=w956, timeout in ms (-1)=0, error in (no error)=w955) -> (element=w960:T24, error out=w954:errorcluster)  [unwired: 2 out]
        n462 = Unbundle By Name(w960) -> ("state"=w958:T17)
        n463 = case shown="Default" w958 {
          selector: w958 -> [_ w965]
          tunnel: [DOCK_SCANNER_sequence_state."initialize" ("state") w965] -> w953
          frame Default {
          }
          frame "stop" {
          }
        }
        n464 = call "wait_on_initialization.vi"("state"=w953) -> ()  [unwired: 11 in]
      }
      frame "stop" {
        # "1. takes so long to close it\nmaybe its not needed?\n2. works faster on server and is needed\nerrors after restart if not closed properly"
        n465 = call <vilib>:"Clear Errors.vi"("error in (no error)"=w971) -> ("error out"=w970:errorcluster)  [unwired: 5 in, 1 out]
        n466 = VISA Close(VISA resource name=w968, error in (no error)=w970) -> (error out=w969:errorcluster)
      }
    }
  }
  n467 = while {
    tunnel: w29 -> [w980]
    shift-right: [w979] -> _
    shift-left: DOCK_PRINTER_sequence_state."initialize" ("DOCK_PRINTER_sequence_state") -> [w978]
    shift-right: [w982] -> w61
    shift-left: w59 -> [w983]
    shift-right: [w977] -> _
    shift-left: _ -> [w976]
    shift-right: [w975] -> _
    shift-left: _ -> [w974]
    stop <- w981 stop-if-true
    # "PRINTER"
    n468 = case shown="\"error\"" w978 {
      tunnel: w983 -> [w992 w1006 w1015 w1023 w1029 w1053]
      tunnel: [w995 w1004 w1021 w1028 w1033 w1049] -> w982
      tunnel: [w993 w1002 w1020 w1027 w1032 DOCK_PRINTER_sequence_state."stop" ("state")] -> w979
      tunnel: [_ _ _ _ _ TRUE] -> w981
      tunnel: w980 -> [w991 w1005 _ _ w1036 _]
      tunnel: [w984 w999 w1012 w1024 w1031 refnum<k5> refnum ("connection ID")] -> w977
      tunnel: w976 -> [_ w999 w1012 w1024 w1031 w1048]
      tunnel: [_ w998 _ _ _ _] -> w975
      tunnel: w974 -> [_ _ w1018 _ _ _]
      frame "initialize" {
        n469 = Unbundle By Name(w991) -> ("main_ini_file.PRINTER IP"=w990:string, "main_ini_file.PRINTER port"=w989:u16, "main_ini_file.PRINTER PC port"=w988:u16)
        n470 = TCP Open Connection(address=w990, remote port or service name=w989, timeout ms (60000)=500, local port=w988, error in (no error)=w992) -> (connection ID=w984:refnum<k5>, error out=w985:errorcluster)
        n471 = Unbundle By Name(w985) -> ("status"=w986:bool)
        n472 = local write "PRINTER_connection_indicator_global"(w986) -> ()
        n473 = call "DOCK_PRINTER_check_for_error.vi"("PRINTER_loop_state_in"=DOCK_PRINTER_sequence_state."get_next_state" ("SQL_EDITOR_sequence_state"), "error_in"=w985) -> ("PRINTER_loop_state_out"=w993:T14, "error_out"=w995:errorcluster)  [unwired: 8 in]
      }
      frame "get_next_state" {
        n474 = Unbundle By Name(w1005) -> ("queue_refnums.PRINTER_queue"=w1007:refnum<queue>, "main_ini_file.PRINTER Keep alive timer [ms]"=w996:i32)
        n475 = Dequeue Element(queue=w1007, timeout in ms (-1)=w996, error in (no error)=w1006) -> (element=w1000:T23, timed out?=w997:bool, error out=w1001:errorcluster)  [unwired: 1 out]
        n476 = case shown="True" w997 {
          tunnel: [w1010 DOCK_PRINTER_sequence_state."keep_alive" ("state")] -> w1003
          tunnel: w1000 -> [w1009 _]
          tunnel: [w1008 _] -> w998
          frame False {
            n477 = Unbundle By Name(w1009) -> ("variable"=w1008:variant, "state"=w1010:T14)
          }
          frame True {
          }
        }
        n478 = call "DOCK_PRINTER_check_for_error.vi"("PRINTER_loop_state_in"=w1003, "error_in"=w1001) -> ("PRINTER_loop_state_out"=w1002:T14, "error_out"=w1004:errorcluster)  [unwired: 8 in]
      }
      frame "send" {
        n479 = Variant To Data(error in=w1015, type="", Variant=w1018) -> (data=w1016:string, error out=w1013:errorcluster)
        n480 = TCP Write(connection ID=w1012, data in=w1016, error in (no error)=w1013) -> (error out=w1014:errorcluster)  [unwired: 1 in, 2 out]
        n481 = call "DOCK_PRINTER_check_for_error.vi"("PRINTER_loop_state_in"=DOCK_PRINTER_sequence_state."get_next_state", "error_in"=w1014) -> ("PRINTER_loop_state_out"=w1020:T14, "error_out"=w1021:errorcluster)  [unwired: 8 in]
      }
      frame "keep_alive" {
        n482 = TCP Write(connection ID=w1024, data in="keepalive", error in (no error)=w1023) -> (error out=w1025:errorcluster)  [unwired: 1 in, 2 out]
        n483 = call "DOCK_PRINTER_check_for_error.vi"("PRINTER_loop_state_in"=DOCK_PRINTER_sequence_state."get_next_state", "error_in"=w1025) -> ("PRINTER_loop_state_out"=w1027:T14, "error_out"=w1028:errorcluster)  [unwired: 8 in]
      }
      frame "error" {
        n484 = disable-structure shown="RUN_TIME_ENGINE==True" {
          disable-tunnel: [w1043 w1044] -> w1034
          disable-tunnel: w1029 -> [w1040 w1045]
          frame condition #0 {
            n485 = call "FGV_DOCK_error_buffer.vi"("thread"=DOCK_thread."PRINTER", "option"=FGV_DOCK_error_buffer."display", "error_in"=w1040) -> ("error_out"=w1043:errorcluster)  [unwired: 7 in, 1 out]
          }
          frame condition #1 (active) {
            n486 = call <vilib>:"Clear Errors.vi"("error in (no error)"=w1045) -> ("error out"=w1044:errorcluster)  [unwired: 5 in, 1 out]
          }
        }
        n487 = Unbundle By Name(w1029) -> ("status"=w1030:bool)
        n488 = Unbundle By Name(w1036) -> ("queue_refnums.PRINTER_queue"=w1035:refnum<queue>)
        n489 = local write "PRINTER_connection_indicator_global"(w1030) -> ()
        n490 = Preview Queue Element(queue=w1035, timeout in ms (-1)=0, error in (no error)=w1034) -> (element=w1039:T23, error out=w1033:errorcluster)  [unwired: 2 out]
        n491 = Unbundle By Name(w1039) -> ("state"=w1037:T14)
        n492 = case shown="Default" w1037 {
          selector: w1037 -> [_ w1047]
          tunnel: [DOCK_PRINTER_sequence_state."initialize" ("state") w1047] -> w1032
          frame Default {
          }
          frame "stop" {
          }
        }
        n493 = call "wait_on_initialization.vi"("state"=w1032) -> ()  [unwired: 11 in]
      }
      frame "stop" {
        n494 = call <vilib>:"Clear Errors.vi"("error in (no error)"=w1053) -> ("error out"=w1050:errorcluster)  [unwired: 5 in, 1 out]
        n495 = TCP Close Connection(connection ID=w1048, error in (no error)=w1050) -> (error out=w1049:errorcluster)  [unwired: 1 in, 1 out]
      }
    }
  }
  n496 = Merge Errors(w73, w71, w70, w61) -> (w72:errorcluster)
  n497 = call "DOCK_destroy_queues.vi"("error_in"=w72, "all_config_info"=w29) -> ("error_out"=w77:errorcluster)  [unwired: 9 in]
  n498 = control-ref of="This VI"() -> (w85:refnum<vi>)
  n499 = call "close_front_panel_in_exe.vi"("error_in"=w77, "vi_reference_in"=w85) -> ("error_out"=w84:errorcluster)  [unwired: 9 in]
  n500 = call <vilib>:"Clear Errors.vi"("error in (no error)"=w84) -> ()  [unwired: 5 in, 2 out]
